vi "运维调试_质控单元.vi"() -> ()   [LabVIEW 2016, in "质控单元.lvlib"]
uses:
  <vilib>/Utility/miscctls.llb/LVPointTypeDef.ctl
  <vilib>/Analysis/6fits.llb/Curve Fitting Criteria.ctl
  <vilib>/Plasmionique/MB Master/MB_Master_Serial/MB_Master_Serial.lvclass
  D:/Program Files (x86)/National Instruments/LabVIEW 2016/vi.lib/Plasmionique/MB Master/MB_Master/MB_Master.lvclass
  <vilib>/Utility/config.llb/Read Key (I32).vi
  <vilib>/Utility/config.llb/Read Key (Double).vi
  <vilib>/Utility/config.llb/Read Key (Boolean).vi
  <vilib>/Utility/config.llb/Read Key (U32).vi
  <vilib>/Utility/config.llb/Write Key (I32).vi
  <vilib>/Utility/config.llb/Write Key (Double).vi
  <vilib>/Utility/config.llb/Write Key (Boolean).vi
  <vilib>/Utility/config.llb/Write Key (U32).vi
  <vilib>/Plasmionique/MB Master/MB Master.lvlib
  <vilib>/ptbypt/NI_PtbyPt.lvlib
  <vilib>/Utility/config.llb/NI_LVConfig.lvlib
  <vilib>/Analysis/NI_AALPro.lvlib
panel:
  in  "柱塞泵4":bool
  in  "CODCr量程选择":enum32{"H", "L", "AUTO"}(ring)
  in  "B 4":dbl caption="B4"
  in  "K 4":dbl caption="K4"
  out "通讯指示灯4":bool
  in  "CODCr选择":bool
  out "CODCr传感器故障报警":bool
  out "CODCr超时报警":bool
  out "CODMn超时报警":bool
  out "总磷总氮超时报警":bool
  out "氨氮进样超时报警":bool
  out "CODMn传感器故障报警":bool
  out "总磷总氮传感器故障报警":bool
  out "氨氮传感器故障报警":bool
  in  "CODCr加标回收启动":bool
  in  "CODCr停止":bool
  in  "CODCr排液":bool
  in  "CODCr调试":bool
  out "CODCr加标回收率":dbl caption="加标回收率" format="%.2f"
  out "CODCr加标体积":dbl caption="加标体积" format="%.3f"
  out "CODCr母液浓度":dbl caption="加标母液浓度" format="%.2f"
  out "CODCr加标水杯定容体积":dbl caption="加标水杯定容体积" format="%.2f"
  out "CODCr加标后水样浓度":dbl caption="加标后水样浓度" format="%.2f"
  out "CODCr加标前水样浓度":dbl caption="加标前水样浓度" format="%.2f"
  out "CODCr检出限":dbl caption="检出限" format="%.2f"
  out "CODCr量程":dbl caption="量程" format="%.2f"
  out "CODCr状态":u16(ring) caption="状态" items=["待机", "润洗", "进样", "等待取液", "排液"]
  out "质控流程中":bool
  out "CODMn质控中断报警":bool
  out "总磷质控中断报警":bool
  out "总氮质控中断报警":bool
  out "氨氮质控中断报警":bool
  in  "报警清除":bool
  in  "CODMn量程选择":enum32{"H", "L", "AUTO"}(ring)
  in  "CODMn加标回收启动":bool
  in  "总磷总氮加标回收启动":bool
  in  "氨氮加标回收启动":bool
  in  "总磷量程选择":enum32{"H", "L", "AUTO"}(ring)=enum."AUTO"
  in  "总氮量程选择":enum32{"H", "L", "AUTO"}(ring)=enum."AUTO"
  in  "氨氮量程选择":enum32{"H", "L", "AUTO"}(ring)=enum."AUTO"
  out "线性值":T1
  out "通讯指示灯3":bool
  out "通讯指示灯2":bool
  out "通讯指示灯1":bool
  in  "CODMn选择":bool
  in  "总磷总氮模块选择":bool
  in  "氨氮模块":bool
  in  "枚举":enum16{"柱塞泵1", "柱塞泵2", "柱塞泵3", "柱塞泵4"}(ring)
  in  "启用":bool
  in  "B 3":dbl caption="B3"
  in  "K 3":dbl caption="K3"
  in  "B 2":dbl caption="B2"
  in  "K 2":dbl caption="K2"
  in  "B":dbl caption="B1"
  in  "K":dbl caption="K1"
  out "r^2":dbl format="%_6g"
  out "拟合方程":string
  in  "实际体积 5":dbl
  in  "标准体积 5":dbl
  in  "实际体积 4":dbl
  in  "标准体积 4":dbl
  in  "实际体积 3":dbl
  in  "实际体积 2":dbl
  in  "实际体积 1":dbl
  in  "标准体积 3":dbl
  in  "标准体积 2":dbl
  in  "标准体积 1":dbl
  in  "读取":bool
  in  "柱塞泵3":bool
  in  "柱塞泵2":bool
  in  "柱塞泵1":bool
  in  "注出体积选择":u16(ring) items=["0.1mL", "0.3mL", "0.5mL", "0.8mL", "1.0mL"]
  out "Serial Config":T2={"baud rate (bps)"=115200, "stop bits"=10, "parity"=0, "flow control"=0, "timeout"=100, "retries"=1} {"stop bits" items=["1.0"=10, "1.5"=15, "2.0"=20]; "parity" items=["None", "Odd", "Even", "Mark", "Space"]; "flow control" items=["None", "XON/XOFF", "RTS/CTS", "XON/XOFF & RTS/CTS", "DTR/DSR", "XON/XOFF & DTR/DSR"]}
  out "VISA Resource":refnum<visa-resource-name>="COM8"
  in  "背隙补偿步数 3":i32 min=0 max=2000
  in  "背隙补偿步数 2":i32 min=0 max=2000
  in  "写入":bool
  in  "背隙补偿步数":i32 min=0 max=2000
  in  "总氮停止":bool
  in  "总氮排液":bool
  in  "总氮调试":bool
  out "总氮加标回收率":dbl caption="加标回收率" format="%.2f"
  out "总氮加标体积":dbl caption="加标体积" format="%.3f"
  out "总氮母液浓度":dbl caption="加标母液浓度" format="%.3f"
  out "总氮加标水杯定容体积":dbl caption="加标水杯定容体积" format="%.2f"
  out "总氮加标后水样浓度":dbl caption="加标后水样浓度" format="%.3f"
  out "总氮加标前水样浓度":dbl caption="加标前水样浓度" format="%.3f"
  out "总氮检出限":dbl caption="检出限" format="%.3f"
  out "总氮量程":dbl caption="量程" format="%.2f"
  out "总氮状态":u16(ring) caption="状态" items=["待机", "润洗", "进样", "等待取液", "排液"]
  in  "返回":bool
  in  "查看":bool
  out "直接启动":bool
  out "常规启动":bool
  out "columns":string[](array[string])
  out "data":T3
  out "COD平行样测完标志":bool
  out "氨氮总磷平行样测完标志":bool
  out "输出簇 2":T4
  out "常规启动 2":bool
  out "直接启动 2":bool
  out "启动模块 2":cluster{"氨氮1":bool, "总磷1":bool, " COD1":bool}
  in  "停止测量":bool
  in  "加标回收":bool
  in  "平行样测试":bool
  in  "CODMn停止":bool
  in  "CODMn排液":bool
  in  "CODMn调试":bool
  in  "总磷停止":bool
  in  "总磷排液":bool
  in  "总磷调试":bool
  out "COD加标回收率":dbl caption="加标回收率" format="%.2f"
  out "COD加标体积":dbl caption="加标体积" format="%.3f"
  out "COD母液浓度":dbl caption="加标母液浓度" format="%.2f"
  out "COD加标水杯定容体积":dbl caption="加标水杯定容体积" format="%.2f"
  out "COD加标后水样浓度":dbl caption="加标后水样浓度" format="%.2f"
  out "COD加标前水样浓度":dbl caption="加标前水样浓度" format="%.2f"
  out "COD检出限":dbl caption="检出限" format="%.2f"
  out "COD量程":dbl caption="量程" format="%.2f"
  out "CODMn状态":u16(ring) caption="状态" items=["待机", "润洗", "进样", "等待取液", "排液"]
  out "总磷加标回收率":dbl caption="加标回收率" format="%.2f"
  out "总磷加标体积":dbl caption="加标体积" format="%.3f"
  out "总磷母液浓度":dbl caption="加标母液浓度" format="%.3f"
  out "总磷加标水杯定容体积":dbl caption="加标水杯定容体积" format="%.2f"
  out "总磷加标后水样浓度":dbl caption="加标后水样浓度" format="%.3f"
  out "总磷加标前水样浓度":dbl caption="加标前水样浓度" format="%.3f"
  out "总磷检出限":dbl caption="检出限" format="%.3f"
  out "总磷量程":dbl caption="量程" format="%.2f"
  out "总磷状态":u16(ring) caption="状态" items=["待机", "润洗", "进样", "等待取液", "排液"]
  out "氨氮加标回收率":dbl caption="加标回收率" format="%.2f"
  out "氨氮加标体积":dbl caption="加标体积" format="%.3f"
  out "氨氮母液浓度":dbl caption="加标母液浓度" format="%.3f"
  out "氨氮加标水杯定容体积":dbl caption="加标水杯定容体积" format="%.2f"
  out "氨氮加标后水样浓度":dbl caption="加标后水样浓度" format="%.3f"
  out "氨氮加标前水样浓度":dbl caption="加标前水样浓度" format="%.3f"
  out "氨氮检出限":dbl caption="检出限" format="%.3f"
  out "氨氮量程":dbl caption="量程" format="%.2f"
  out "氨氮状态":u16(ring) caption="状态" items=["待机", "润洗", "进样", "等待取液", "排液"]
  in  "氨氮停止":bool
  in  "氨氮排液":bool
  in  "氨氮调试":bool
  # "状态显示区"
  # "参数配置区"
  # "2000步等于1mL\n100步等于0.05mL\n20步等于0.01mL\n2步等于0.001mL\n（初始默认100步）"
  # "辅助计算区"
  # "柱塞泵调试区"
  # "CODCr质控参数"
  # "%"
  # "mL"
  # "mg/L"
  # "mL"
  # "mg/L"
  # "mg/L"
  # "mg/L"
  # "mg/L"
  # "总氮质控参数"
  # "%"
  # "mL"
  # "mg/L"
  # "mL"
  # "mg/L"
  # "mg/L"
  # "mg/L"
  # "mg/L"
  # "CODMn质控参数"
  # "%"
  # "mL"
  # "mg/L"
  # "mL"
  # "mg/L"
  # "mg/L"
  # "mg/L"
  # "mg/L"
  # "总磷质控参数"
  # "%"
  # "mL"
  # "mg/L"
  # "mL"
  # "mg/L"
  # "mg/L"
  # "mg/L"
  # "mg/L"
  # "氨氮质控参数"
  # "%"
  # "mL"
  # "mg/L"
  # "mL"
  # "mg/L"
  # "mg/L"
  # "mg/L"
  # "mg/L"
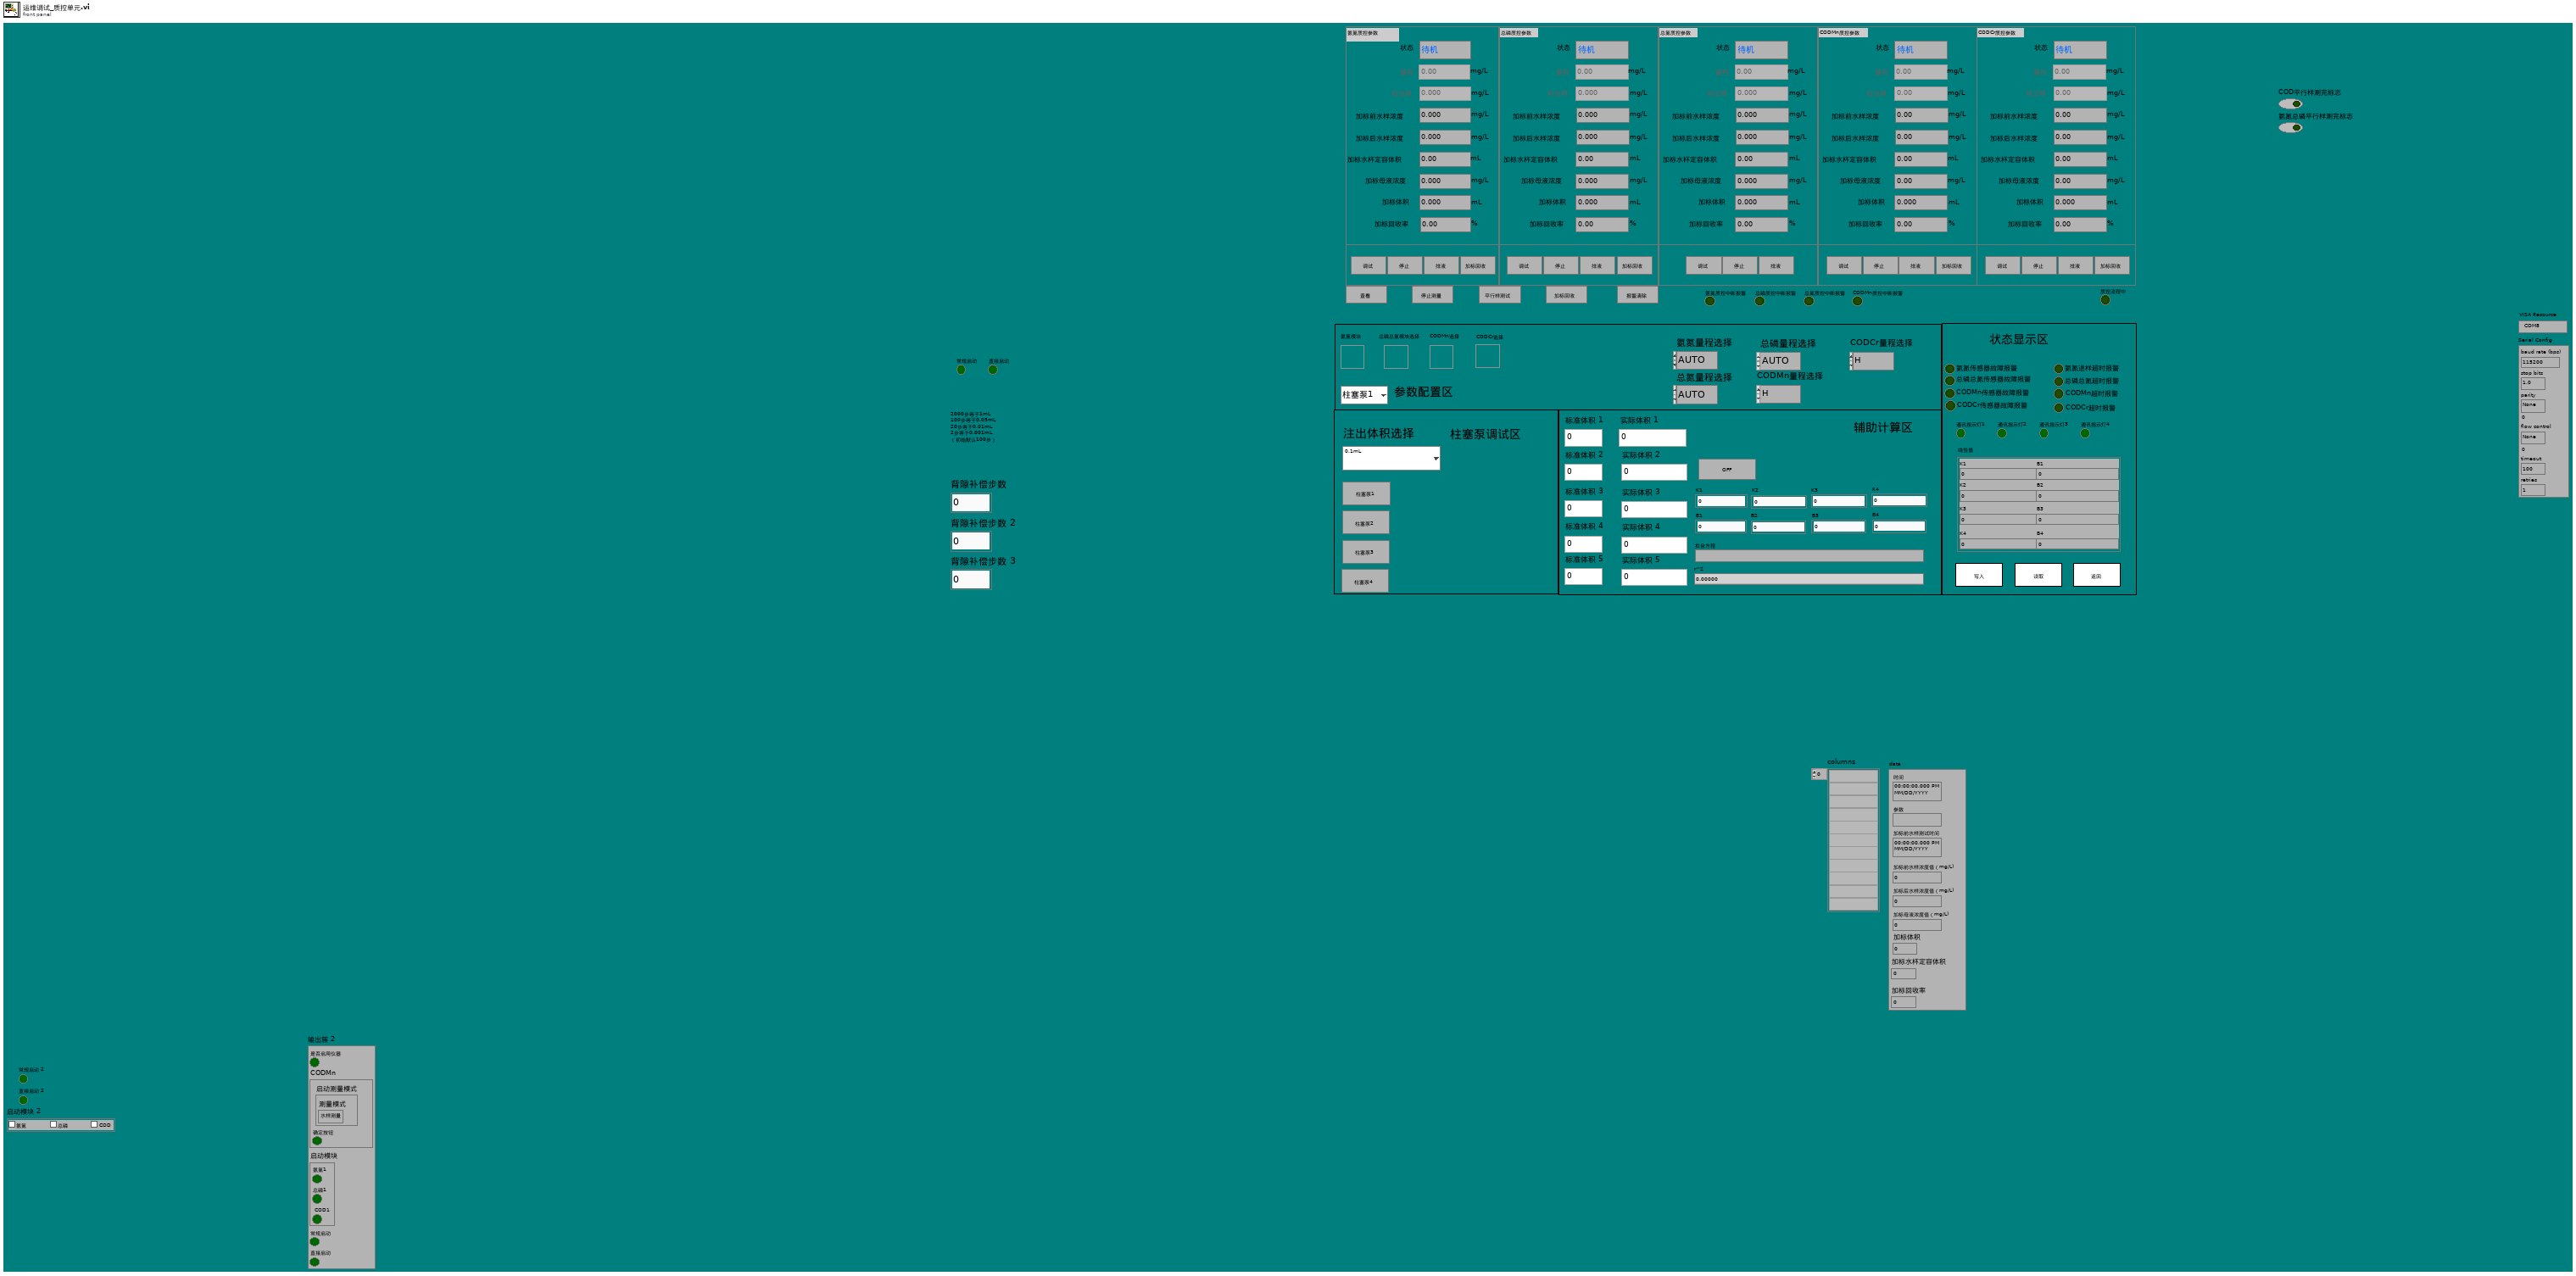
[diagram p1: front panel]
types:
  T1 = cluster{"K1":sgl, "B1":sgl, "K2":sgl, "B2":sgl, "K3":sgl, "B3":sgl, "K4":sgl, "B4":sgl}
  T2 = cluster{"baud rate (bps)":u32, "stop bits":u16, "parity":u16, "flow control":u16, "timeout":u32, "retries":i32}
  T3 = cluster{"时间":timestamp, "参数":string, "加标前水样测试时间":timestamp, "加标前水样浓度值（mg/L)":sgl, "加标后水样浓度值（mg/L)":sgl, "加标母液浓度值（mg/L)":sgl, "加标体积":dbl, "加标水杯定容体积":dbl, "加标回收率":dbl}
  T4 = cluster{"是否启用仪器":bool, "CODMn":cluster{"启动测量模式":cluster{"测量模式":enum16{"水样测量", "标样核查", "加标回收", "平行样", "校零", "校标"}}, "确定按钮":bool}, "启动模块":cluster{"氨氮1":bool, "总磷1":bool, " COD1":bool}, "常规启动":bool, "直接启动":bool}
  T5 = typedef "LVPointTypeDef.ctl" = cluster{"Horizontal":i16, "Vertical":i16}
  T6 = cluster{"量程":dbl, "检出限":dbl, "加标前水样浓度":dbl, "加标后水样浓度":dbl, "加标水杯定容体积":dbl, "加标母液浓度":dbl, "加标体积":dbl, "加标回收率":dbl}
  T7 = cluster{"因子编码":u32, "单位":u16, "标样参考值":sgl, "水样数据时间":timestamp, "水样实测值":sgl, "水样数据标识":string, "标样数据时间":timestamp, "标样实测值":sgl, "标样数据标识":string, "空白数据时间":timestamp, "空白实测值":sgl, "空白数据标识":string, "零点核查数据时间":timestamp, "零点核查实测值":sgl, "零点核查数据标识":string, "跨度核查数据时间":timestamp, "跨度核查实测值":sgl, "跨度核查数据标识":string, "加标回收数据时间":timestamp, "加标回收实测值":sgl, "加标回收数据标识":string, "平行样数据时间":timestamp, "平行样实测值":sgl, "平行样数据标识":string}
  T8 = cluster{"因子编码":u32, "单位":u16, "标样参考值":sgl, "水样数据时间":timestamp, "水样实测值":sgl, "水样数据标识":string, "标样数据时间":timestamp, "标样实测值":sgl, "标样数据标识":string, "空白数据时间":timestamp, "空白实测值":sgl, "空白数据标识":string, "零点核查数据时间":timestamp, "零点核查实测值":sgl, "零点核查数据标识":string, "跨度核查数据时间":timestamp, "跨度核查实测值":sgl, "跨度核查数据标识":string, "加标回收数据时间":timestamp, "加标回收实测值":sgl, "加标回收数据标识":string, "平行样数据时间":timestamp, "平行样实测值":sgl, "平行样数据标识":string, "F0":sgl, "F1":sgl, "F2":sgl, "F3":sgl, "F4":sgl, "F5":sgl, "F6":sgl, "F7":sgl, "温度":sgl, "湿度":sgl, "X值":sgl}
  T9 = enum8{"Enabled", "Disabled", "Disabled and Grayed Out"}
  T10 = typedef "NI_AALPro.lvlib/Curve Fitting Criteria.ctl" = u16
  T11 = typedef "NI_LVConfig.lvlib/Config Data RefNum.ctl" = refnum<k1>
  T12 = cluster{"是否启用仪器":bool, "CODMn":cluster{"启动测量模式":cluster{"测量模式":enum16{"水样测量", "标样核查", "加标回收", "平行样", "校零", "校标"}}, "确定按钮":bool}, "启动模块":cluster{"氨氮":bool, "总磷":bool, "总氮":bool, "CODMn":bool, "CODCr":bool}, "常规启动":bool, "直接启动":bool}
  T13 = cluster{"是否启用仪器":bool, "CODMn":cluster{"启动测量模式":cluster{"测量模式":enum16{"水样测量", "标样核查", "加标回收", "平行样", "校零", "校标"}}, "确定按钮":bool}, "启动模块":cluster{"氨氮":bool, "总磷":bool, "总氮":bool, "COD":bool}, "常规启动":bool, "直接启动":bool}
  T14 = cluster{"命令":string, cluster{"starting address":u16, "holding register value":u16}}
  T15 = cluster{"氨氮":bool, "总磷":bool, "总氮":bool, "CODMn":bool, "CODCr":bool}
  T16 = enum32{"Bad", "Idle", "Run top level", "Running"}
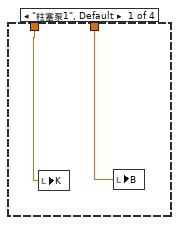
[diagram p3: hidden frame]
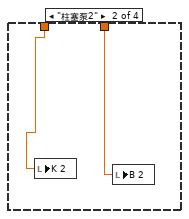
[diagram p4: hidden frame]
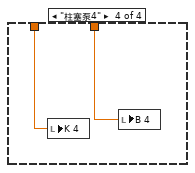
[diagram p5: hidden frame]
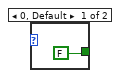
[diagram p8: hidden frame]
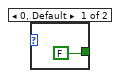
[diagram p9: hidden frame]
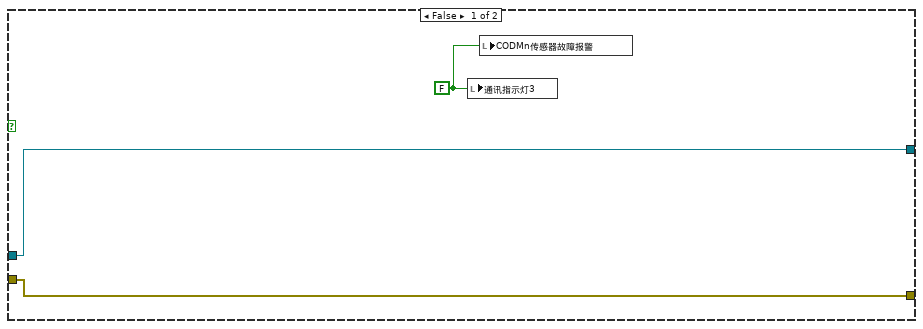
[diagram p10: hidden frame]
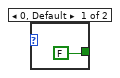
[diagram p11: hidden frame]
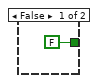
[diagram p12: hidden frame]
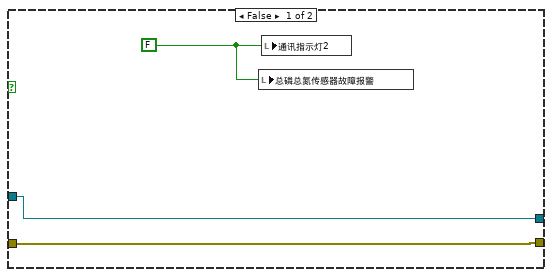
[diagram p13: hidden frame]
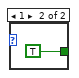
[diagram p14: hidden frame]
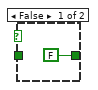
[diagram p15: hidden frame]
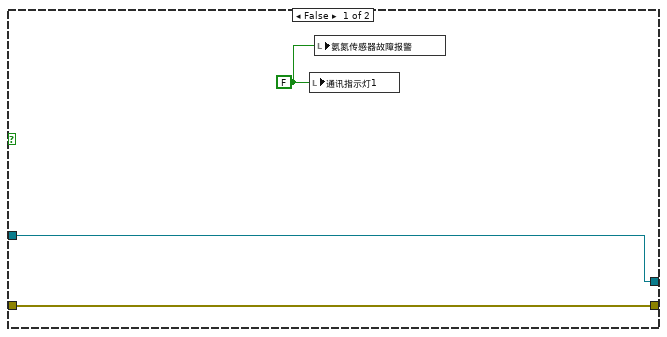
[diagram p16: hidden frame]
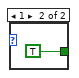
[diagram p17: hidden frame]
diagram:
  w21 = T2 {"baud rate (bps)"=115200, "stop bits"=10, "parity"=0, "flow control"=0, "timeout"=500, "retries"=1} ("Serial Config")
  w22 = refnum<visa-resource-name> "COM8" ("VISA Resource")
  n1 = global write "串口参数全局.vi" "Serial Config"(w21) -> ()
  n2 = control-ref of="总氮加标回收率"() -> (w36:refnum<vi>)
  n3 = control-ref of="总氮加标体积"() -> (w37:refnum<vi>)
  n4 = control-ref of="总氮加标水杯定容体积"() -> (w39:refnum<vi>)
  n5 = control-ref of="总氮加标后水样浓度"() -> (w40:refnum<vi>)
  n6 = control-ref of="总氮母液浓度"() -> (w38:refnum<vi>)
  n7 = global write "串口参数全局.vi" "VISA Resource"(w22) -> ()
  n8 = control-ref of="总氮检出限"() -> (w42:refnum<vi>)
  n9 = control-ref of="总氮加标前水样浓度"() -> (w41:refnum<vi>)
  n10 = control-ref of="总氮量程"() -> (w43:refnum<vi>)
  n11 = call <vilib>:"Open Serial Session.vi"("Mode (RTU)"=enum16{"RTU", "ASCII"}."RTU", "Slave ID"=u8 10, "Serial Config"=w21, "VISA Resource"=w22) -> ("Error out"=w54:errorcluster, "MB_Serial session"=w55:refnum<class "MB_Master_Serial.lvclass">)  [unwired: 6 in]
  n12 = control-ref of="COD加标水杯定容体积"() -> (w60:refnum<vi>)
  n13 = control-ref of="COD加标前水样浓度"() -> (w62:refnum<vi>)
  n14 = control-ref of="COD加标后水样浓度"() -> (w61:refnum<vi>)
  n15 = property on="窗格" class="Pane"("Origin"=T5 {"Horizontal"=0, "Vertical"=0} ("原点")) -> ()  [unwired: 2 in, 2 out]
  n16 = property on="窗格" class="Pane"("Origin"=T5 {"Horizontal"=0, "Vertical"=0} ("原点")) -> ()  [unwired: 2 in, 2 out]
  n17 = call "质控参数读取.vi"("section"="氨氮质控参数") -> ("error out"=w85:errorcluster, "参数"=w104:T6)  [unwired: 9 in]
  n18 = while {
    tunnel: w55 -> [w162]
    tunnel: w54 -> [w161]
    tunnel: [w128] -> w53
    tunnel: [w129] -> w23
    stop <- FALSE stop-if-true
    n19 = local read "CODCr加标前水样浓度"() -> (w126:dbl)
    n20 = global read "水样浓度全局.vi" "CODCr加标前水样浓度"() -> (w127:dbl)
    n21 = global read "质控测完标志全局 1.vi" "总磷总氮平行样测完标志"() -> (→"氨氮总磷平行样测完标志":bool)
    n22 = local read "氨氮模块"() -> (w135:bool)
    n23 = case shown="真" w135 {
      tunnel: w162 -> [w262 w282]
      tunnel: w161 -> [w261 w281]
      tunnel: [w262 w270] -> w139
      tunnel: [w261 w269] -> w137
      frame False {
        w260 = FALSE ("通讯指示灯1")
        n24 = local write "通讯指示灯1"(w260) -> ()
        n25 = local write "氨氮传感器故障报警"(w260) -> ()
      }
      frame True {
        n26 = property class="MB_Master_Serial"(reference=w282, "Properties:Slave ID"=u8 1 ("Slave ID")) -> (reference out=w277:refnum<class "MB_Master_Serial.lvclass">)  [unwired: 1 in, 1 out]
        n27 = call <vilib>:"Read Holding Registers.vi"("error in (no error)"=w281, "quantity"=u16 5, "starting address"=u16 100, "MB session in"=w277) -> ("error out"=w269:errorcluster, "Registers"=w278:u16[], "MB session out"=w270:refnum<class "MB_Master_Serial.lvclass">)  [unwired: 5 in]
        n28 = Index Array(array=w278, index #2=4 ("索引"), index #3=5 ("索引")) -> (element #1=w263:u16, element #2=w274:u16, element #3=w265:u16)  [unwired: 1 in]
        "氨氮状态" <- w263
        n29 = Unbundle By Name(w269) -> ("status"=w268:bool)
        n30 = case shown="0, 默认" w265 {
          tunnel: [FALSE TRUE] -> w264
          frame 0, Default {
          }
          frame 1 {
          }
        }
        "氨氮进样超时报警" <- w264
        n31 = global write "氨氮加标回收状态全局变量.vi" "氨氮状态"(w263) -> ()
        n32 = Not(x=w268) -> (.not. x?=→"通讯指示灯1":bool)
        n33 = Equal?(x=w274, y=u16 1) -> (x = y?=w271:bool)
        n34 = case shown="假" w271 {
          tunnel: w271 -> [_ w286]
          tunnel: [FALSE w286] -> w272
          frame False {
          }
          frame True {
          }
        }
        "氨氮传感器故障报警" <- w272
      }
    }
    n35 = global read "质控测完标志全局 1.vi" "氨氮加标回收测完标志"() -> (w148:bool)
    n36 = global read "质控测完标志全局 1.vi" "总磷加标回收测完标志"() -> (w140:bool)
    n37 = global read "质控测完标志全局 1.vi" "COD平行样测完标志"() -> (→"COD平行样测完标志":bool)
    n38 = global read "水样浓度全局.vi" "COD加标前水样浓度"() -> (w156:dbl)
    n39 = local read "总氮加标前水样浓度"() -> (w143:dbl)
    n40 = global read "水样浓度全局.vi" "氨氮加标前水样浓度"() -> (w160:dbl)
    n41 = global read "水样浓度全局.vi" "总磷加标前水样浓度"() -> (w158:dbl)
    n42 = local read "COD加标前水样浓度"() -> (w155:dbl)
    n43 = global read "水样浓度全局.vi" "总氮加标前水样浓度"() -> (w142:dbl)
    n44 = local read "氨氮加标前水样浓度"() -> (w159:dbl)
    n45 = local read "总磷加标前水样浓度"() -> (w157:dbl)
    n46 = global read "质控测完标志全局 1.vi" "COD加标回收测完标志"() -> (w123:bool)
    n47 = global read "质控测完标志全局 1.vi" "CODCr加标回收测完标志"() -> (w117:bool)
    n48 = global read "质控测完标志全局 1.vi" "总氮加标回收测完标志"() -> (w120:bool)
    n49 = Wait (ms)(milliseconds to wait=u32 1000 ("等待时间（毫秒）")) -> ()  [unwired: 1 out]
    n50 = Not Equal?(x=w127, y=w126) -> (x != y?=w125:bool)
    n51 = Not Equal?(x=w160, y=w159) -> (x != y?=w154:bool)
    n52 = Not Equal?(x=w158, y=w157) -> (x != y?=w152:bool)
    n53 = Not Equal?(x=w156, y=w155) -> (x != y?=w151:bool)
    n54 = Not Equal?(x=w142, y=w143) -> (x != y?=w141:bool)
    n55 = call <vilib>:"Boolean Crossing PtByPt.vi"("direction"=enum16{"either", "false-true", "true-false"}."false-true", "input"=w148) -> ("crossing"=w147:bool)  [unwired: 1 in]
    n56 = call <vilib>:"Boolean Crossing PtByPt.vi"("direction"=enum16{"either", "false-true", "true-false"}."false-true", "input"=w140) -> ("crossing"=w144:bool)  [unwired: 1 in]
    n57 = call <vilib>:"Boolean Crossing PtByPt.vi"("direction"=enum16{"either", "false-true", "true-false"}."false-true", "input"=w123) -> ("crossing"=w122:bool)  [unwired: 1 in]
    n58 = call <vilib>:"Boolean Crossing PtByPt.vi"("direction"=enum16{"either", "false-true", "true-false"}."false-true", "input"=w120) -> ("crossing"=w119:bool)  [unwired: 1 in]
    n59 = call <vilib>:"Boolean Crossing PtByPt.vi"("direction"=enum16{"either", "false-true", "true-false"}."false-true", "input"=w117) -> ("crossing"=w116:bool)  [unwired: 1 in]
    n60 = case shown="真" w147 {
      frame False {
      }
      frame True {
        n61 = flat-sequence {
          frame #0 {
            n62 = global read "VAR氨氮全局变量.vi" "测量数据区"() -> (w338:T7)
            n63 = Unbundle By Name(w338) -> ("加标回收实测值"=w339:sgl)
            n64 = property on="氨氮加标后水样浓度" class="DigNum (严格)"("Val(Sgnl)"=w339) -> ()  [unwired: 2 in, 2 out]
          }
          frame #1 {
            n65 = Wait (ms)(milliseconds to wait=u32 500 ("等待时间（毫秒）")) -> ()  [unwired: 1 out]
          }
          frame #2 {
            n66 = global read "VAR氨氮全局变量.vi" "测量数据区"() -> (w344:T7)
            n67 = local read "氨氮加标水杯定容体积"() -> (w350:dbl)
            n68 = global read "水样浓度全局.vi" "氨氮加标前水样浓度"() -> (w354:dbl)
            n69 = Unbundle By Name(w344) -> ("加标回收数据时间"=w347:timestamp)
            n70 = Unbundle By Name(w344) -> ("加标回收实测值"=w353:sgl)
            n71 = Unbundle By Name(w344) -> ("水样数据时间"=w345:timestamp)
            n72 = local read "氨氮加标回收率"() -> (w349:dbl)
            n73 = local read "氨氮母液浓度"() -> (w352:dbl)
            n74 = local read "氨氮加标体积"() -> (w351:dbl)
            n75 = Bundle By Name(cluster=T3 {"时间"=timestamp(0 s since 1904-01-01), "参数"="", "加标前水样测试时间"=timestamp(0 s since 1904-01-01), "加标前水样浓度值（mg/L)"=0.0, "加标后水样浓度值（mg/L)"=0.0, "加标母液浓度值（mg/L)"=0.0, "加标体积"=0.0, "加标水杯定容体积"=0.0, "加标回收率"=0.0} ("data"), "时间"=w347, "参数"="氨氮加标回收率" ("table"), "加标前水样测试时间"=w345, "加标前水样浓度值（mg/L)"=w354, "加标后水样浓度值（mg/L)"=w353, "加标母液浓度值（mg/L)"=w352, "加标体积"=w351, "加标水杯定容体积"=w350, "加标回收率"=w349) -> (w341:T3)
            n76 = local read "columns"() -> (w342:string[])
            n77 = local write "data"(w341) -> ()
            n78 = call "数据写入databaseZK.vi"("data"=w341, "columns"=w342, "table"="加标回收率") -> ()  [unwired: 8 in, 1 out]
          }
        }
      }
    }
    n79 = case shown="真" w144 {
      frame False {
      }
      frame True {
        n80 = flat-sequence {
          frame #0 {
            n81 = global read "VAR总磷总氮全局变量.vi" "总磷测量数据区"() -> (w321:T8)
            n82 = Unbundle By Name(w321) -> ("加标回收实测值"=w322:sgl)
            n83 = property on="总磷加标后水样浓度" class="DigNum (严格)"("Val(Sgnl)"=w322) -> ()  [unwired: 2 in, 2 out]
          }
          frame #1 {
            n84 = Wait (ms)(milliseconds to wait=u32 500 ("等待时间（毫秒）")) -> ()  [unwired: 1 out]
          }
          frame #2 {
            n85 = global read "VAR总磷总氮全局变量.vi" "总磷测量数据区"() -> (w327:T8)
            n86 = Unbundle By Name(w327) -> ("加标回收数据时间"=w330:timestamp)
            n87 = Unbundle By Name(w327) -> ("加标回收实测值"=w328:sgl)
            n88 = Unbundle By Name(w327) -> ("水样数据时间"=w329:timestamp)
            n89 = local read "总磷加标水杯定容体积"() -> (w334:dbl)
            n90 = local read "总磷加标回收率"() -> (w333:dbl)
            n91 = local read "总磷母液浓度"() -> (w336:dbl)
            n92 = local read "总磷加标体积"() -> (w335:dbl)
            n93 = global read "水样浓度全局.vi" "总磷加标前水样浓度"() -> (w337:dbl)
            n94 = Bundle By Name(cluster=T3 {"时间"=timestamp(0 s since 1904-01-01), "参数"="", "加标前水样测试时间"=timestamp(0 s since 1904-01-01), "加标前水样浓度值（mg/L)"=0.0, "加标后水样浓度值（mg/L)"=0.0, "加标母液浓度值（mg/L)"=0.0, "加标体积"=0.0, "加标水杯定容体积"=0.0, "加标回收率"=0.0} ("data"), "时间"=w330, "参数"="总磷加标回收率" ("table"), "加标前水样测试时间"=w329, "加标前水样浓度值（mg/L)"=w337, "加标后水样浓度值（mg/L)"=w328, "加标母液浓度值（mg/L)"=w336, "加标体积"=w335, "加标水杯定容体积"=w334, "加标回收率"=w333) -> (w324:T3)
            "data" <- w324
            n95 = local read "columns"() -> (w325:string[])
            n96 = call "数据写入databaseZK.vi"("data"=w324, "columns"=w325, "table"="加标回收率") -> ()  [unwired: 8 in, 1 out]
          }
        }
      }
    }
    n97 = case shown="真" w122 {
      frame False {
      }
      frame True {
        n98 = flat-sequence {
          frame #0 {
            n99 = global read "COD浓度全局变量.vi" "COD浓度（mg/L)"() -> (w306:dbl)
            n100 = property on="COD加标后水样浓度" class="DigNum (严格)"("Val(Sgnl)"=w306) -> ()  [unwired: 2 in, 2 out]
          }
          frame #1 {
            n101 = Wait (ms)(milliseconds to wait=u32 500 ("等待时间（毫秒）")) -> ()  [unwired: 1 out]
          }
          frame #2 {
            n102 = local read "COD加标水杯定容体积"() -> (w316:dbl)
            n103 = global read "水样浓度全局.vi" "COD加标前水样浓度"() -> (w320:dbl)
            n104 = global read "COD浓度全局变量.vi" "COD浓度（mg/L)"() -> (w319:dbl)
            n105 = global read "COD测量模式全局.vi" "加标回收启动时间"() -> (w312:timestamp)
            n106 = global read "COD测量模式全局.vi" "水样启动时间"() -> (w311:timestamp)
            n107 = local read "COD加标回收率"() -> (w315:dbl)
            n108 = local read "COD母液浓度"() -> (w318:dbl)
            n109 = local read "COD加标体积"() -> (w317:dbl)
            n110 = Bundle By Name(cluster=T3 {"时间"=timestamp(0 s since 1904-01-01), "参数"="", "加标前水样测试时间"=timestamp(0 s since 1904-01-01), "加标前水样浓度值（mg/L)"=0.0, "加标后水样浓度值（mg/L)"=0.0, "加标母液浓度值（mg/L)"=0.0, "加标体积"=0.0, "加标水杯定容体积"=0.0, "加标回收率"=0.0} ("data"), "时间"=w312, "参数"="CODMn加标回收率" ("table"), "加标前水样测试时间"=w311, "加标前水样浓度值（mg/L)"=w320, "加标后水样浓度值（mg/L)"=w319, "加标母液浓度值（mg/L)"=w318, "加标体积"=w317, "加标水杯定容体积"=w316, "加标回收率"=w315) -> (w308:T3)
            n111 = local read "columns"() -> (w309:string[])
            n112 = local write "data"(w308) -> ()
            n113 = call "数据写入databaseZK.vi"("data"=w308, "columns"=w309, "table"="加标回收率") -> ()  [unwired: 8 in, 1 out]
          }
        }
      }
    }
    n114 = case shown="真" w119 {
      frame False {
      }
      frame True {
        n115 = flat-sequence {
          frame #0 {
            n116 = global read "VAR总磷总氮全局变量.vi" "总氮测量数据区"() -> (w288:T8)
            n117 = Unbundle By Name(w288) -> ("加标回收实测值"=w287:sgl)
            n118 = property on="总氮加标后水样浓度" class="DigNum (严格)"("Val(Sgnl)"=w287) -> ()  [unwired: 2 in, 2 out]
          }
          frame #1 {
            n119 = Wait (ms)(milliseconds to wait=u32 500 ("等待时间（毫秒）")) -> ()  [unwired: 1 out]
          }
          frame #2 {
            n120 = global read "VAR总磷总氮全局变量.vi" "总氮测量数据区"() -> (w298:T8)
            n121 = global read "VAR总磷总氮全局变量.vi" "总氮测量数据区"() -> (w294:T8)
            n122 = global read "VAR总磷总氮全局变量.vi" "总氮测量数据区"() -> (w304:T8)
            n123 = local read "总氮加标水杯定容体积"() -> (w300:dbl)
            n124 = global read "水样浓度全局.vi" "总氮加标前水样浓度"() -> (w305:dbl)
            n125 = Unbundle By Name(w298) -> ("加标回收数据时间"=w295:timestamp)
            n126 = Unbundle By Name(w304) -> ("加标回收实测值"=w303:sgl)
            n127 = Unbundle By Name(w294) -> ("水样数据时间"=w293:timestamp)
            n128 = local read "总氮加标回收率"() -> (w299:dbl)
            n129 = local read "总氮母液浓度"() -> (w302:dbl)
            n130 = local read "总氮加标体积"() -> (w301:dbl)
            n131 = Bundle By Name(cluster=T3 {"时间"=timestamp(0 s since 1904-01-01), "参数"="", "加标前水样测试时间"=timestamp(0 s since 1904-01-01), "加标前水样浓度值（mg/L)"=0.0, "加标后水样浓度值（mg/L)"=0.0, "加标母液浓度值（mg/L)"=0.0, "加标体积"=0.0, "加标水杯定容体积"=0.0, "加标回收率"=0.0} ("data"), "时间"=w295, "参数"="总氮加标回收率" ("table"), "加标前水样测试时间"=w293, "加标前水样浓度值（mg/L)"=w305, "加标后水样浓度值（mg/L)"=w303, "加标母液浓度值（mg/L)"=w302, "加标体积"=w301, "加标水杯定容体积"=w300, "加标回收率"=w299) -> (w290:T3)
            n132 = local read "columns"() -> (w291:string[])
            n133 = local write "data"(w290) -> ()
            n134 = call "数据写入databaseZK.vi"("data"=w290, "columns"=w291, "table"="加标回收率") -> ()  [unwired: 8 in, 1 out]
          }
        }
      }
    }
    n135 = case shown="真" w116 {
      frame False {
      }
      frame True {
        n136 = flat-sequence {
          frame #0 {
            n137 = global read "CODcr全局变量.vi" "测量数据区"() -> (w166:T7)
            n138 = Unbundle By Name(w166) -> ("加标回收实测值"=w165:sgl)
            n139 = property on="CODCr加标后水样浓度" class="DigNum (严格)"("Val(Sgnl)"=w165) -> ()  [unwired: 2 in, 2 out]
          }
          frame #1 {
            n140 = Wait (ms)(milliseconds to wait=u32 500 ("等待时间（毫秒）")) -> ()  [unwired: 1 out]
          }
          frame #2 {
            n141 = global read "CODcr全局变量.vi" "测量数据区"() -> (w174:T7)
            n142 = global read "CODcr全局变量.vi" "测量数据区"() -> (w173:T7)
            n143 = global read "CODcr全局变量.vi" "测量数据区"() -> (w172:T7)
            n144 = local read "CODCr加标水杯定容体积"() -> (w169:dbl)
            n145 = local read "CODCr加标回收率"() -> (w168:dbl)
            n146 = local read "CODCr母液浓度"() -> (w171:dbl)
            n147 = local read "CODCr加标体积"() -> (w170:dbl)
            n148 = global read "水样浓度全局.vi" "CODCr加标前水样浓度"() -> (w183:dbl)
            n149 = Unbundle By Name(w172) -> ("加标回收数据时间"=w179:timestamp)
            n150 = Unbundle By Name(w174) -> ("加标回收实测值"=w182:sgl)
            n151 = Unbundle By Name(w173) -> ("水样数据时间"=w178:timestamp)
            n152 = Bundle By Name(cluster=T3 {"时间"=timestamp(0 s since 1904-01-01), "参数"="", "加标前水样测试时间"=timestamp(0 s since 1904-01-01), "加标前水样浓度值（mg/L)"=0.0, "加标后水样浓度值（mg/L)"=0.0, "加标母液浓度值（mg/L)"=0.0, "加标体积"=0.0, "加标水杯定容体积"=0.0, "加标回收率"=0.0} ("data"), "时间"=w179, "参数"="CODCr加标回收率" ("table"), "加标前水样测试时间"=w178, "加标前水样浓度值（mg/L)"=w183, "加标后水样浓度值（mg/L)"=w182, "加标母液浓度值（mg/L)"=w171, "加标体积"=w170, "加标水杯定容体积"=w169, "加标回收率"=w168) -> (w175:T3)
            n153 = local read "columns"() -> (w176:string[])
            n154 = local write "data"(w175) -> ()
            n155 = call "数据写入databaseZK.vi"("data"=w175, "columns"=w176, "table"="加标回收率") -> ()  [unwired: 8 in, 1 out]
          }
        }
      }
    }
    n156 = Compound Arithmetic op=OR ("复合运算")(w154, w152, w151, w141, w125) -> (w153:bool)
    n157 = case shown="真" w153 {
      frame False {
      }
      frame True {
        n158 = global read "水样浓度全局.vi" "CODCr加标前水样浓度"() -> (w355:dbl)
        n159 = property on="CODCr加标前水样浓度" class="DigNum (严格)"("Val(Sgnl)"=w355) -> ()  [unwired: 2 in, 2 out]
        n160 = global read "水样浓度全局.vi" "COD加标前水样浓度"() -> (w357:dbl)
        n161 = global read "水样浓度全局.vi" "总氮加标前水样浓度"() -> (w356:dbl)
        n162 = global read "水样浓度全局.vi" "总磷加标前水样浓度"() -> (w358:dbl)
        n163 = global read "水样浓度全局.vi" "氨氮加标前水样浓度"() -> (w359:dbl)
        n164 = property on="总氮加标前水样浓度" class="DigNum (严格)"("Val(Sgnl)"=w356) -> ()  [unwired: 2 in, 2 out]
        n165 = property on="COD加标前水样浓度" class="DigNum (严格)"("Val(Sgnl)"=w357) -> ()  [unwired: 2 in, 2 out]
        n166 = property on="总磷加标前水样浓度" class="DigNum (严格)"("Val(Sgnl)"=w358) -> ()  [unwired: 2 in, 2 out]
        n167 = property on="氨氮加标前水样浓度" class="DigNum (严格)"("Val(Sgnl)"=w359) -> ()  [unwired: 2 in, 2 out]
      }
    }
    n168 = local read "总磷总氮模块选择"() -> (w134:bool)
    n169 = case shown="真" w134 {
      tunnel: w139 -> [w236 w250]
      tunnel: [w236 w249] -> w138
      tunnel: w137 -> [w235 w248]
      tunnel: [w235 w246] -> w136
      frame False {
        w234 = FALSE ("通讯指示灯2")
        n170 = local write "总磷总氮传感器故障报警"(w234) -> ()
        n171 = local write "通讯指示灯2"(w234) -> ()
      }
      frame True {
        n172 = property class="MB_Master_Serial"(reference=w250, "Properties:Slave ID"=u8 2 ("Slave ID")) -> (reference out=w252:refnum<class "MB_Master_Serial.lvclass">)  [unwired: 1 in, 1 out]
        n173 = call <vilib>:"Read Holding Registers.vi"("error in (no error)"=w248, "quantity"=u16 5, "starting address"=u16 100, "MB session in"=w252) -> ("error out"=w246:errorcluster, "Registers"=w255:u16[], "MB session out"=w249:refnum<class "MB_Master_Serial.lvclass">)  [unwired: 5 in]
        n174 = Unbundle By Name(w246) -> ("status"=w247:bool)
        n175 = Index Array(array=w255, index #2=4 ("索引")) -> (element #1=w239:u16, element #2=w242:u16, element #3=w237:u16)  [unwired: 2 in]
        "总氮状态" <- w239
        "总磷状态" <- w239
        n176 = case shown="0, 默认" w237 {
          tunnel: [FALSE TRUE] -> w238
          frame 0, Default {
          }
          frame 1 {
          }
        }
        "总磷总氮超时报警" <- w238
        n177 = Not(x=w247) -> (.not. x?=→"通讯指示灯2":bool)
        n178 = Equal?(x=w242, y=u16 1) -> (x = y?=w240:bool)
        n179 = case shown="真" w240 {
          tunnel: w240 -> [_ w259]
          tunnel: [FALSE w259] -> w241
          frame False {
          }
          frame True {
          }
        }
        "总磷总氮传感器故障报警" <- w241
        n180 = global write "氨氮加标回收状态全局变量.vi" "总磷状态"(w239) -> ()
        n181 = global write "氨氮加标回收状态全局变量.vi" "总氮状态"(w239) -> ()
      }
    }
    n182 = local read "CODMn选择"() -> (w133:bool)
    n183 = case shown="真" w133 {
      tunnel: [w210 w225] -> w130
      tunnel: w138 -> [w210 w217]
      tunnel: w136 -> [w209 w216]
      tunnel: [w209 w214] -> w131
      frame False {
        w208 = FALSE ("通讯指示灯3")
        n184 = local write "通讯指示灯3"(w208) -> ()
        n185 = local write "CODMn传感器故障报警"(w208) -> ()
      }
      frame True {
        n186 = property class="MB_Master_Serial"(reference=w217, "Properties:Slave ID"=u8 3 ("Slave ID")) -> (reference out=w228:refnum<class "MB_Master_Serial.lvclass">)  [unwired: 1 in, 1 out]
        n187 = call <vilib>:"Read Holding Registers.vi"("error in (no error)"=w216, "quantity"=u16 5, "starting address"=u16 100, "MB session in"=w228) -> ("error out"=w214:errorcluster, "Registers"=w224:u16[], "MB session out"=w225:refnum<class "MB_Master_Serial.lvclass">)  [unwired: 5 in]
        n188 = Unbundle By Name(w214) -> ("status"=w215:bool)
        n189 = Index Array(array=w224, index #2=4 ("索引")) -> (element #1=w222:u16, element #2=w219:u16, element #3=w211:u16)  [unwired: 2 in]
        "CODMn状态" <- w222
        n190 = global write "氨氮加标回收状态全局变量.vi" "COD状态"(w222) -> ()
        n191 = Not(x=w215) -> (.not. x?=→"通讯指示灯3":bool)
        n192 = case shown="1" w211 {
          tunnel: [FALSE TRUE] -> w212
          frame 0, Default {
          }
          frame 1 {
          }
        }
        "CODMn超时报警" <- w212
        n193 = Equal?(x=w219, y=u16 1) -> (x = y?=w221:bool)
        n194 = case shown="真" w221 {
          tunnel: w221 -> [_ w233]
          tunnel: [FALSE w233] -> w218
          frame False {
          }
          frame True {
          }
        }
        "CODMn传感器故障报警" <- w218
      }
    }
    n195 = local read "CODCr选择"() -> (w132:bool)
    n196 = case shown="真" w132 {
      tunnel: w131 -> [w184 w202]
      tunnel: w130 -> [w185 w201]
      tunnel: [w185 w194] -> w129
      tunnel: [w184 w193] -> w128
      frame False {
      }
      frame True {
        n197 = property class="MB_Master_Serial"(reference=w201, error in=w202, "Properties:Slave ID"=u8 4 ("Slave ID")) -> (reference out=w196:refnum<class "MB_Master_Serial.lvclass">, error out=w195:errorcluster)
        n198 = call <vilib>:"Read Holding Registers.vi"("error in (no error)"=w195, "quantity"=u16 5, "starting address"=u16 100, "MB session in"=w196) -> ("error out"=w193:errorcluster, "Registers"=w198:u16[], "MB session out"=w194:refnum<class "MB_Master_Serial.lvclass">)  [unwired: 5 in]
        n199 = Unbundle By Name(w193) -> ("status"=w192:bool)
        n200 = Index Array(array=w198, index #2=4 ("索引")) -> (element #1=w190:u16, element #2=w187:u16, element #3=w189:u16)  [unwired: 2 in]
        "CODCr状态" <- w190
        n201 = global write "氨氮加标回收状态全局变量.vi" "CODCr状态"(w190) -> ()
        n202 = Not(x=w192) -> (.not. x?=→"通讯指示灯4":bool)
        n203 = case shown="1" w187 {
          tunnel: [FALSE TRUE] -> w186
          frame 0, Default {
          }
          frame 1 {
          }
        }
        "CODCr传感器故障报警" <- w186
        n204 = case shown="1" w189 {
          tunnel: [FALSE TRUE] -> w188
          frame 0, Default {
          }
          frame 1 {
          }
        }
        "CODCr超时报警" <- w188
      }
    }
  }
  n205 = Build Array(w43, w42, w41, w40, w39, w38, w37, w36) -> (w35:refnum<vi>[])
  n206 = while {
    stop <- FALSE stop-if-true
    n207 = global read "质控测完标志全局 1.vi" "氨氮质控流程中"() -> (w370:bool)
    n208 = global read "质控测完标志全局 1.vi" "COD质控流程中"() -> (w362:bool)
    n209 = global read "质控测完标志全局 1.vi" "总氮质控流程中"() -> (w366:bool)
    n210 = global read "质控中断报警全局.vi" "CODMn中断报警"() -> (→"CODMn质控中断报警":bool)
    n211 = global read "质控中断报警全局.vi" "氨氮中断报警"() -> (→"氨氮质控中断报警":bool)
    n212 = global read "质控中断报警全局.vi" "总氮中断报警"() -> (→"总氮质控中断报警":bool)
    n213 = Wait (ms)(milliseconds to wait=u32 100 ("等待时间（毫秒）")) -> ()  [unwired: 1 out]
    n214 = global read "质控中断报警全局.vi" "总磷中断报警"() -> (→"总磷质控中断报警":bool)
    n215 = local read "CODMn状态"() -> (w387:u16)
    n216 = global read "质控测完标志全局 1.vi" "质控流程中"() -> (w373:bool)
    "质控流程中" <- w373
    n217 = local read "总氮状态"() -> (w385:u16)
    n218 = local read "氨氮状态"() -> (w401:u16)
    n219 = local read "总磷状态"() -> (w392:u16)
    n220 = Not Equal To 0?(x=w385) -> (x != 0?=w384:bool)
    n221 = Not Equal To 0?(x=w401) -> (x != 0?=w400:bool)
    n222 = Not Equal To 0?(x=w392) -> (x != 0?=w394:bool)
    n223 = Not Equal To 0?(x=w387) -> (x != 0?=w391:bool)
    n224 = Select(t=T9."Disabled and Grayed Out" ("禁用"), s=w400, f=T9."Enabled") -> (s? t:f=w397:T9)
    n225 = Select(t=T9."Disabled and Grayed Out" ("禁用"), s=w394, f=T9."Enabled") -> (s? t:f=w393:T9)
    n226 = Select(t=T9."Disabled and Grayed Out" ("禁用"), s=w391, f=T9."Enabled") -> (s? t:f=w388:T9)
    n227 = Select(t=T9."Disabled and Grayed Out" ("禁用"), s=w370, f=T9."Enabled") -> (s? t:f=w368:T9)
    n228 = Select(t=T9."Disabled and Grayed Out" ("禁用"), s=w362, f=T9."Enabled") -> (s? t:f=w360:T9)
    n229 = Select(t=T9."Disabled and Grayed Out" ("禁用"), s=w366, f=T9."Enabled") -> (s? t:f=w364:T9)
    n230 = Select(t=T9."Disabled and Grayed Out" ("禁用"), s=w384, f=T9."Enabled") -> (s? t:f=w381:T9)
    n231 = Select(t=T9."Disabled and Grayed Out" ("禁用"), s=w373, f=T9."Enabled") -> (s? t:f=w372:T9)
    n232 = property on="氨氮加标回收启动" class="Bool"("DisabledEnum"=w368) -> ()  [unwired: 2 in, 2 out]
    n233 = property on="氨氮调试" class="Bool"("DisabledEnum"=w397) -> ()  [unwired: 2 in, 2 out]
    n234 = property on="总磷调试" class="Bool"("DisabledEnum"=w393) -> ()  [unwired: 2 in, 2 out]
    n235 = property on="COD调试" class="Bool"("DisabledEnum"=w388) -> ()  [unwired: 2 in, 2 out]
    n236 = property on="总磷总氮加标回收启动" class="Bool"("DisabledEnum"=w364) -> ()  [unwired: 2 in, 2 out]
    n237 = property on="CODMn加标回收启动" class="Bool"("DisabledEnum"=w360) -> ()  [unwired: 2 in, 2 out]
    n238 = property on="加标回收" class="Bool"("DisabledEnum"=w372) -> ()  [unwired: 2 in, 2 out]
    n239 = property on="总氮调试" class="Bool"("DisabledEnum"=w381) -> ()  [unwired: 2 in, 2 out]
    n240 = case shown="真" "启用" {
      frame False {
      }
      frame True {
        w419 = T10 0 items=["最小二乘", "最小绝对残差", "Bisquare"] ("method")
        n241 = Build Array("标准体积 1", "标准体积 2", "标准体积 3", "标准体积 4", "标准体积 5") -> (w416:dbl[])
        n242 = Build Array("实际体积 1", "实际体积 2", "实际体积 3", "实际体积 4", "实际体积 5") -> (w417:dbl[])
        n243 = call "线性公式质控用.vi"("标液浓度"=w416, "模型"=enum32{"线性", "多项式"}."线性", "监测浓度"=w417, "启用"=bool[] [TRUE, TRUE, TRUE, TRUE, TRUE], "method"=w419) -> ("拟合方程"=→"拟合方程":string, "r^2"=→"r^2":dbl, "slope"=w405:dbl, "intercept"=w404:dbl)  [unwired: 6 in, 1 out]
        n244 = case shown="\"柱塞泵3\"" "枚举" {
          tunnel: w405 -> [w423 w426 w427 w430]
          tunnel: w404 -> [w424 w425 w428 w429]
          frame "柱塞泵1", Default {
            n245 = local write "K"(w423) -> ()
            n246 = local write "B"(w424) -> ()
          }
          frame "柱塞泵2" {
            n247 = local write "K 2"(w426) -> ()
            n248 = local write "B 2"(w425) -> ()
          }
          frame "柱塞泵3" {
            n249 = local write "K 3"(w427) -> ()
            n250 = local write "B 3"(w428) -> ()
          }
          frame "柱塞泵4" {
            n251 = local write "K 4"(w430) -> ()
            n252 = local write "B 4"(w429) -> ()
          }
        }
      }
    }
  }
  n253 = control-ref of="总磷加标水杯定容体积"() -> (w69:refnum<vi>)
  n254 = control-ref of="氨氮加标水杯定容体积"() -> (w111:refnum<vi>)
  n255 = Unbundle By Name(w104) -> ("量程"=→"氨氮量程":dbl, "检出限"=→"氨氮检出限":dbl, "加标前水样浓度"=→"氨氮加标前水样浓度":dbl, "加标后水样浓度"=→"氨氮加标后水样浓度":dbl, "加标水杯定容体积"=→"氨氮加标水杯定容体积":dbl, "加标母液浓度"=→"氨氮母液浓度":dbl, "加标体积"=→"氨氮加标体积":dbl, "加标回收率"=→"氨氮加标回收率":dbl)
  n256 = control-ref of="总磷加标前水样浓度"() -> (w71:refnum<vi>)
  n257 = control-ref of="总磷加标后水样浓度"() -> (w70:refnum<vi>)
  n258 = control-ref of="氨氮加标前水样浓度"() -> (w112:refnum<vi>)
  n259 = control-ref of="氨氮加标后水样浓度"() -> (w108:refnum<vi>)
  n260 = control-ref of="COD加标回收率"() -> (w57:refnum<vi>)
  n261 = control-ref of="CODCr加标后水样浓度"() -> (w6:refnum<vi>)
  n262 = control-ref of="CODCr加标回收率"() -> (w2:refnum<vi>)
  n263 = control-ref of="CODCr加标前水样浓度"() -> (w7:refnum<vi>)
  n264 = control-ref of="CODCr加标水杯定容体积"() -> (w5:refnum<vi>)
  n265 = control-ref of="COD母液浓度"() -> (w59:refnum<vi>)
  n266 = control-ref of="COD加标体积"() -> (w58:refnum<vi>)
  n267 = control-ref of="CODCr检出限"() -> (w8:refnum<vi>)
  n268 = control-ref of="CODCr母液浓度"() -> (w4:refnum<vi>)
  n269 = control-ref of="CODCr量程"() -> (w9:refnum<vi>)
  n270 = control-ref of="CODCr加标体积"() -> (w3:refnum<vi>)
  n271 = call "质控参数读取.vi"("section"="总磷质控参数", "error in (no error)"=w85) -> ("error out"=w82:errorcluster, "参数"=w94:T6)  [unwired: 8 in]
  n272 = control-ref of="总磷加标回收率"() -> (w67:refnum<vi>)
  n273 = control-ref of="氨氮加标回收率"() -> (w106:refnum<vi>)
  n274 = control-ref of="COD检出限"() -> (w63:refnum<vi>)
  n275 = control-ref of="总磷母液浓度"() -> (w68:refnum<vi>)
  n276 = control-ref of="总磷加标体积"() -> (w66:refnum<vi>)
  n277 = control-ref of="氨氮母液浓度"() -> (w110:refnum<vi>)
  n278 = control-ref of="氨氮加标体积"() -> (w107:refnum<vi>)
  n279 = control-ref of="COD量程"() -> (w64:refnum<vi>)
  n280 = control-ref of="总磷检出限"() -> (w72:refnum<vi>)
  n281 = control-ref of="氨氮检出限"() -> (w113:refnum<vi>)
  n282 = control-ref of="总磷量程"() -> (w73:refnum<vi>)
  n283 = control-ref of="氨氮量程"() -> (w114:refnum<vi>)
  n284 = Build Array(w9, w8, w7, w6, w5, w4, w3, w2) -> (w1:refnum<vi>[])
  n285 = Obtain Notifier(name (unnamed)="采配水Process" ("名称（未命名）"), notification data type=FALSE) -> (notifier out=w48:refnum<notifier>)  [unwired: 2 in, 2 out]
  n286 = Build Array(w64, w63, w62, w61, w60, w59, w58, w57) -> (w56:refnum<vi>[])
  n287 = Build Array(w73, w72, w71, w70, w69, w68, w66, w67) -> (w65:refnum<vi>[])
  n288 = Build Array(w114, w113, w112, w108, w111, w110, w107, w106) -> (w109:refnum<vi>[])
  n289 = Unbundle By Name(w94) -> ("量程"=→"总磷量程":dbl, "检出限"=→"总磷检出限":dbl, "加标前水样浓度"=→"总磷加标前水样浓度":dbl, "加标后水样浓度"=→"总磷加标后水样浓度":dbl, "加标水杯定容体积"=→"总磷加标水杯定容体积":dbl, "加标母液浓度"=→"总磷母液浓度":dbl, "加标体积"=→"总磷加标体积":dbl, "加标回收率"=→"总磷加标回收率":dbl)
  n290 = call "质控参数读取.vi"("section"="COD质控参数", "error in (no error)"=w82) -> ("error out"=w33:errorcluster, "参数"=w84:T6)  [unwired: 8 in]
  n291 = Unbundle By Name(w84) -> ("量程"=→"COD量程":dbl, "检出限"=→"COD检出限":dbl, "加标前水样浓度"=→"COD加标前水样浓度":dbl, "加标后水样浓度"=→"COD加标后水样浓度":dbl, "加标水杯定容体积"=→"COD加标水杯定容体积":dbl, "加标母液浓度"=→"COD母液浓度":dbl, "加标体积"=→"COD加标体积":dbl, "加标回收率"=→"COD加标回收率":dbl)
  n292 = call "质控参数读取.vi"("section"="总氮质控参数", "error in (no error)"=w33) -> ("error out"=w18:errorcluster, "参数"=w32:T6)  [unwired: 8 in]
  n293 = Unbundle By Name(w32) -> ("量程"=→"总氮量程":dbl, "检出限"=→"总氮检出限":dbl, "加标前水样浓度"=→"总氮加标前水样浓度":dbl, "加标后水样浓度"=→"总氮加标后水样浓度":dbl, "加标水杯定容体积"=→"总氮加标水杯定容体积":dbl, "加标母液浓度"=→"总氮母液浓度":dbl, "加标体积"=→"总氮加标体积":dbl, "加标回收率"=→"总氮加标回收率":dbl)
  n294 = flat-sequence {
    frame #0 {
      w442 = "质控模块量程选择" ("section")
      w434 = "质控模块选择" ("section")
      w508 = "质控线性参数" ("section")
      w526 = "质控背隙补偿" ("section")
      n295 = call <vilib>:"Application Directory.vi"() -> ("Application Directory"=w532:path)
      n296 = Build Path(base path=w532, name or relative path="data\\Set.ini" ("名称或相对路径")) -> (appended path=w530:path)
      n297 = call <vilib>:"Open Config Data.vi"("configuration file path"=w530) -> ("error out"=w528:errorcluster, "refnum"=w529:T11)  [unwired: 8 in, 1 out]
      n298 = call-poly <vilib>:"Read Key.vi"("section"=w526, "error in (no error)"=w528, "key"="背隙值1", "refnum"=w529) -> ("error out"=w523:errorcluster, "value"=w518:i32, "refnum out"=w525:T11)  [unwired: 4 in, 1 out]
      n299 = local write "背隙补偿步数"(w518) -> ()
      n300 = call-poly <vilib>:"Read Key.vi"("section"=w526, "error in (no error)"=w523, "key"="背隙值2", "refnum"=w525) -> ("error out"=w521:errorcluster, "value"=w519:i32, "refnum out"=w522:T11)  [unwired: 4 in, 1 out]
      n301 = local write "背隙补偿步数 2"(w519) -> ()
      n302 = call-poly <vilib>:"Read Key.vi"("section"=w526, "error in (no error)"=w521, "key"="背隙值3", "refnum"=w522) -> ("error out"=w515:errorcluster, "value"=w517:i32, "refnum out"=w516:T11)  [unwired: 4 in, 1 out]
      n303 = local write "背隙补偿步数 3"(w517) -> ()
      n304 = call-poly <vilib>:"Read Key.vi"("section"=w508, "error in (no error)"=w515, "key"="标准体积1", "refnum"=w516) -> ("error out"=w511:errorcluster, "value"=w513:dbl, "refnum out"=w512:T11)  [unwired: 4 in, 1 out]
      n305 = local write "标准体积 1"(w513) -> ()
      n306 = call-poly <vilib>:"Read Key.vi"("section"=w508, "error in (no error)"=w511, "key"="标准体积2", "refnum"=w512) -> ("error out"=w509:errorcluster, "value"=w502:dbl, "refnum out"=w510:T11)  [unwired: 4 in, 1 out]
      n307 = local write "标准体积 2"(w502) -> ()
      n308 = call-poly <vilib>:"Read Key.vi"("section"=w508, "error in (no error)"=w509, "key"="标准体积3", "refnum"=w510) -> ("error out"=w506:errorcluster, "value"=w501:dbl, "refnum out"=w507:T11)  [unwired: 4 in, 1 out]
      n309 = local write "标准体积 3"(w501) -> ()
      n310 = call-poly <vilib>:"Read Key.vi"("section"=w508, "error in (no error)"=w506, "key"="标准体积4", "refnum"=w507) -> ("error out"=w504:errorcluster, "value"=w486:dbl, "refnum out"=w505:T11)  [unwired: 4 in, 1 out]
      n311 = local write "标准体积 4"(w486) -> ()
      n312 = Build Array("时间" ("table"), "参数" ("table"), "加标前水样测试时间" ("table"), "加标前水样浓度值" ("元素"), "加标后水样浓度值" ("元素"), "加标母液浓度值" ("元素"), "加标体积" ("元素"), "加标水杯定容体积" ("元素"), "加标回收率" ("元素")) -> (→"columns":string[])
      n313 = call-poly <vilib>:"Read Key.vi"("section"=w508, "error in (no error)"=w504, "key"="标准体积5", "refnum"=w505) -> ("error out"=w495:errorcluster, "value"=w485:dbl, "refnum out"=w496:T11)  [unwired: 4 in, 1 out]
      n314 = local write "标准体积 5"(w485) -> ()
      n315 = call-poly <vilib>:"Read Key.vi"("section"=w508, "error in (no error)"=w495, "key"="实际体积1", "refnum"=w496) -> ("error out"=w493:errorcluster, "value"=w484:dbl, "refnum out"=w494:T11)  [unwired: 4 in, 1 out]
      n316 = local write "实际体积 1"(w484) -> ()
      n317 = call-poly <vilib>:"Read Key.vi"("section"=w508, "error in (no error)"=w493, "key"="实际体积2", "refnum"=w494) -> ("error out"=w491:errorcluster, "value"=w483:dbl, "refnum out"=w492:T11)  [unwired: 4 in, 1 out]
      n318 = local write "实际体积 2"(w483) -> ()
      n319 = call-poly <vilib>:"Read Key.vi"("section"=w508, "error in (no error)"=w491, "key"="实际体积3", "refnum"=w492) -> ("error out"=w489:errorcluster, "value"=w480:dbl, "refnum out"=w490:T11)  [unwired: 4 in, 1 out]
      n320 = local write "实际体积 3"(w480) -> ()
      n321 = call-poly <vilib>:"Read Key.vi"("section"=w508, "error in (no error)"=w489, "key"="实际体积4", "refnum"=w490) -> ("error out"=w487:errorcluster, "value"=w479:dbl, "refnum out"=w488:T11)  [unwired: 4 in, 1 out]
      n322 = local write "实际体积 4"(w479) -> ()
      n323 = call-poly <vilib>:"Read Key.vi"("section"=w508, "error in (no error)"=w487, "key"="实际体积5", "refnum"=w488) -> ("error out"=w474:errorcluster, "value"=w478:dbl, "refnum out"=w475:T11)  [unwired: 4 in, 1 out]
      n324 = local write "实际体积 5"(w478) -> ()
      n325 = call-poly <vilib>:"Read Key.vi"("section"="质控手动体积选择", "error in (no error)"=w474, "key"="手动体积选择" ("section"), "refnum"=w475) -> ("error out"=w469:errorcluster, "value"=w471:i32, "refnum out"=w470:T11)  [unwired: 4 in, 1 out]
      n326 = local write "注出体积选择"(w471) -> ()
      n327 = call-poly <vilib>:"Read Key.vi"("section"=w434, "error in (no error)"=w469, "key"="模块1" ("section"), "refnum"=w470) -> ("error out"=w467:errorcluster, "value"=w459:bool, "refnum out"=w468:T11)  [unwired: 4 in, 1 out]
      n328 = call-poly <vilib>:"Read Key.vi"("section"=w434, "error in (no error)"=w467, "key"="模块2" ("section"), "refnum"=w468) -> ("error out"=w465:errorcluster, "value"=w460:bool, "refnum out"=w466:T11)  [unwired: 4 in, 1 out]
      n329 = local write "氨氮模块"(w459) -> ()
      n330 = local write "总磷总氮模块选择"(w460) -> ()
      n331 = call-poly <vilib>:"Read Key.vi"("section"=w434, "error in (no error)"=w465, "key"="模块3" ("section"), "refnum"=w466) -> ("error out"=w436:errorcluster, "value"=w461:bool, "refnum out"=w437:T11)  [unwired: 4 in, 1 out]
      n332 = local write "CODMn选择"(w461) -> ()
      n333 = call-poly <vilib>:"Read Key.vi"("section"=w434, "error in (no error)"=w436, "key"="模块4", "refnum"=w437) -> ("error out"=w432:errorcluster, "value"=w431:bool, "refnum out"=w433:T11)  [unwired: 4 in, 1 out]
      n334 = local write "CODCr选择"(w431) -> ()
      n335 = call-poly <vilib>:"Read Key.vi"("section"=w442, "error in (no error)"=w432, "key"="氨氮" ("section"), "refnum"=w433) -> ("error out"=w457:errorcluster, "value"=w448:u32, "refnum out"=w458:T11)  [unwired: 4 in, 1 out]
      n336 = local write "氨氮量程选择"(w448) -> ()
      n337 = call-poly <vilib>:"Read Key.vi"("section"=w442, "error in (no error)"=w457, "key"="总氮" ("section"), "refnum"=w458) -> ("error out"=w455:errorcluster, "value"=w447:u32, "refnum out"=w456:T11)  [unwired: 4 in, 1 out]
      n338 = local write "总氮量程选择"(w447) -> ()
      n339 = call-poly <vilib>:"Read Key.vi"("section"=w442, "error in (no error)"=w455, "key"="总磷" ("section"), "refnum"=w456) -> ("error out"=w453:errorcluster, "value"=w446:u32, "refnum out"=w454:T11)  [unwired: 4 in, 1 out]
      n340 = local write "总磷量程选择"(w446) -> ()
      n341 = call-poly <vilib>:"Read Key.vi"("section"=w442, "error in (no error)"=w453, "key"="CODMn" ("section"), "refnum"=w454) -> ("error out"=w443:errorcluster, "value"=w445:u32, "refnum out"=w444:T11)  [unwired: 4 in, 1 out]
      n342 = local write "CODMn量程选择"(w445) -> ()
      n343 = call-poly <vilib>:"Read Key.vi"("section"=w442, "error in (no error)"=w443, "key"="CODCr" ("section"), "refnum"=w444) -> ("error out"=w439:errorcluster, "value"=w440:u32, "refnum out"=w438:T11)  [unwired: 4 in, 1 out]
      n344 = local write "CODCr量程选择"(w440) -> ()
      n345 = call <vilib>:"Close Config Data.vi"("error in (no error)"=w439, "refnum"=w438) -> ()  [unwired: 8 in, 2 out]
    }
  }
  n346 = Obtain Queue(name (unnamed)="采配水" ("名称（未命名）"), element data type=cluster{"命令":string, "数据":variant} {"命令"="", "数据"=variant}) -> (queue out=w45:refnum<queue>)  [unwired: 3 in, 2 out]
  n347 = while {
    tunnel: w109 -> [w549]
    tunnel: w65 -> [w548]
    tunnel: w56 -> [w543]
    tunnel: w48 -> [w547]
    tunnel: w45 -> [w546]
    tunnel: w35 -> [w545]
    tunnel: w1 -> [w544]
    stop <- FALSE stop-if-true
    # "氨氮站号是1，总磷总氮站号是2，COD站号是3"
    n348 = event shown="[34] \"CODCr母液浓度\", \"CODCr加标水杯定容体积\", \"CODCr加标前水样浓度\", \"CODCr检出限\", \"CODCr量程\", \"CODCr加标后水样浓度\": 值改变" {
      selector: _ -> [_ _ _ _ _ _ _ _ _ _ _ _ _ _ _ _ _ _ _ _ _ _ _ _ _ _ _ _ _ _ _ _ _ _ _ _ _ _ _ _ _ _ _ _ _ _ _ _]
      dyn-events: _ -> [_ _ _ _ _ _ _ _ _ _ _ _ _ _ _ _ _ _ _ _ _ _ _ _ _ _ _ _ _ _ _ _ _ _ _ _ _ _ _ _ _ _ _ _ _ _ _ _]
      timeout: _ -> [_ _ _ _ _ _ _ _ _ _ _ _ _ _ _ _ _ _ _ _ _ _ _ _ _ _ _ _ _ _ _ _ _ _ _ _ _ _ _ _ _ _ _ _ _ _ _ _]
      tunnel: w549 -> [_ _ _ _ _ _ _ _ _ _ _ _ _ _ _ _ _ _ _ _ _ _ _ _ _ _ _ _ _ _ w916 _ _ _ _ w1013 _ _ _ _ _ _ _ _ _ _ _ _]
      tunnel: w548 -> [_ _ _ _ _ _ _ _ _ _ _ _ _ _ _ _ _ _ _ _ _ _ _ _ _ _ _ _ _ _ _ w930 _ _ _ w1010 _ _ _ _ _ _ _ _ _ _ _ _]
      tunnel: w543 -> [_ _ _ _ _ _ _ _ _ _ _ _ _ _ _ _ _ _ _ _ _ _ _ _ _ _ _ _ _ _ _ _ _ w968 _ w1009 _ _ _ _ _ _ _ _ _ _ _ _]
      tunnel: w547 -> [_ _ _ _ _ _ _ _ _ _ _ _ _ _ _ _ _ _ _ _ _ _ _ _ _ _ _ _ _ _ _ _ _ _ _ _ _ _ w1042 _ _ _ _ _ w1203 w1234 _ _]
      tunnel: w546 -> [_ _ _ _ _ _ _ _ _ _ _ _ _ _ _ _ _ _ _ _ _ _ _ _ _ _ _ _ _ _ _ _ _ _ _ _ _ _ _ _ _ _ _ _ _ w1231 _ _]
      tunnel: w545 -> [_ _ _ _ _ _ _ _ _ _ _ _ _ _ _ _ _ _ _ _ _ _ _ _ _ _ _ _ _ _ _ _ w948 _ _ w1006 _ _ _ _ _ _ _ _ _ _ _ _]
      tunnel: [_ _ _ _ _ _ _ _ _ _ _ _ _ _ _ _ _ _ _ _ _ _ _ _ _ w841 w882 w889 w896 w903 _ _ _ _ _ _ _ _ _ w1072 _ _ _ _ _ _ _ _] -> _
      tunnel: w544 -> [_ _ _ _ _ _ _ _ _ _ _ _ _ _ _ _ _ _ _ _ _ _ _ _ _ _ _ _ _ _ _ _ _ _ w986 w1005 _ _ _ _ _ _ _ _ _ _ _ _]
      event Timeout {
        n349 = event-data() -> ()  [unwired: 1 in, 3 out]
      }
      event "氨氮量程", "氨氮检出限", "氨氮加标前水样浓度", "氨氮加标水杯定容体积", "氨氮母液浓度", "氨氮加标后水样浓度": Mouse Down {
        n350 = event-data() -> ("CtlRef"=w554:refnum<vi>)  [unwired: 1 in, 7 out]
        n351 = property class="DigNum (严格)"(reference=w554) -> (reference out=w552:refnum<vi>, "Value"=w553:dbl)  [unwired: 1 in, 1 out]
        n352 = call "数字键盘.vi"("OldNumber"=w553) -> ("NewNumber"=w551:sgl)
        n353 = property class="DigNum (严格)"(reference=w552, "Val(Sgnl)"=w551) -> ()  [unwired: 1 in, 2 out]
      }
      event "总磷母液浓度", "总磷加标水杯定容体积", "总磷加标后水样浓度", "总磷加标前水样浓度", "总磷检出限", "总磷量程": Mouse Down {
        n354 = event-data() -> ("CtlRef"=w558:refnum<vi>)  [unwired: 1 in, 7 out]
        n355 = property class="DigNum (严格)"(reference=w558) -> (reference out=w556:refnum<vi>, "Value"=w557:dbl)  [unwired: 1 in, 1 out]
        n356 = call "数字键盘.vi"("OldNumber"=w557) -> ("NewNumber"=w555:sgl)
        n357 = property class="DigNum (严格)"(reference=w556, "Val(Sgnl)"=w555) -> ()  [unwired: 1 in, 2 out]
      }
      event "总氮母液浓度", "总氮加标水杯定容体积", "总氮加标后水样浓度", "总氮加标前水样浓度", "总氮检出限", "总氮量程": Mouse Down {
        n358 = event-data() -> ("CtlRef"=w562:refnum<vi>)  [unwired: 1 in, 7 out]
        n359 = property class="DigNum (严格)"(reference=w562) -> (reference out=w560:refnum<vi>, "Value"=w561:dbl)  [unwired: 1 in, 1 out]
        n360 = call "数字键盘.vi"("OldNumber"=w561) -> ("NewNumber"=w559:sgl)
        n361 = property class="DigNum (严格)"(reference=w560, "Val(Sgnl)"=w559) -> ()  [unwired: 1 in, 2 out]
      }
      event "COD母液浓度", "COD加标水杯定容体积", "COD加标后水样浓度", "COD加标前水样浓度", "COD检出限", "COD量程": Mouse Down {
        n362 = event-data() -> ("CtlRef"=w566:refnum<vi>)  [unwired: 1 in, 7 out]
        n363 = property class="DigNum (严格)"(reference=w566) -> (reference out=w564:refnum<vi>, "Value"=w565:dbl)  [unwired: 1 in, 1 out]
        n364 = call "数字键盘.vi"("OldNumber"=w565) -> ("NewNumber"=w563:sgl)
        n365 = property class="DigNum (严格)"(reference=w564, "Val(Sgnl)"=w563) -> ()  [unwired: 1 in, 2 out]
      }
      event "CODCr检出限", "CODCr量程", "CODCr加标前水样浓度", "CODCr加标后水样浓度", "CODCr加标水杯定容体积", "CODCr母液浓度": Mouse Down {
        n366 = event-data() -> ("CtlRef"=w567:refnum<vi>)  [unwired: 1 in, 7 out]
        n367 = property class="DigNum (严格)"(reference=w567) -> (reference out=w569:refnum<vi>, "Value"=w570:dbl)  [unwired: 1 in, 1 out]
        n368 = call "数字键盘.vi"("OldNumber"=w570) -> ("NewNumber"=w568:sgl)
        n369 = property class="DigNum (严格)"(reference=w569, "Val(Sgnl)"=w568) -> ()  [unwired: 1 in, 2 out]
      }
      event "背隙补偿步数": Mouse Down {
        n370 = event-data() -> ()  [unwired: 1 in, 8 out]
        n371 = local read "背隙补偿步数"() -> (w572:i32)
        n372 = call "数字键盘.vi"("OldNumber"=w572) -> ("NewNumber"=w571:sgl)
        n373 = local write "背隙补偿步数"(w571) -> ()
      }
      event "标准体积 1": Mouse Down {
        n374 = event-data() -> ()  [unwired: 1 in, 8 out]
        n375 = local read "标准体积 1"() -> (w574:dbl)
        n376 = call "数字键盘.vi"("OldNumber"=w574) -> ("NewNumber"=w573:sgl)
        n377 = local write "标准体积 1"(w573) -> ()
      }
      event "标准体积 2": Mouse Down {
        n378 = event-data() -> ()  [unwired: 1 in, 8 out]
        n379 = local read "标准体积 2"() -> (w576:dbl)
        n380 = call "数字键盘.vi"("OldNumber"=w576) -> ("NewNumber"=w575:sgl)
        n381 = local write "标准体积 2"(w575) -> ()
      }
      event "标准体积 3": Mouse Down {
        n382 = event-data() -> ()  [unwired: 1 in, 8 out]
        n383 = local read "标准体积 3"() -> (w578:dbl)
        n384 = call "数字键盘.vi"("OldNumber"=w578) -> ("NewNumber"=w577:sgl)
        n385 = local write "标准体积 3"(w577) -> ()
      }
      event "标准体积 4": Mouse Down {
        n386 = event-data() -> ()  [unwired: 1 in, 8 out]
        n387 = local read "标准体积 4"() -> (w580:dbl)
        n388 = call "数字键盘.vi"("OldNumber"=w580) -> ("NewNumber"=w579:sgl)
        n389 = local write "标准体积 4"(w579) -> ()
      }
      event "标准体积 5": Mouse Down {
        n390 = event-data() -> ()  [unwired: 1 in, 8 out]
        n391 = local read "标准体积 5"() -> (w582:dbl)
        n392 = call "数字键盘.vi"("OldNumber"=w582) -> ("NewNumber"=w581:sgl)
        n393 = local write "标准体积 5"(w581) -> ()
      }
      event "实际体积 1": Mouse Down {
        n394 = event-data() -> ()  [unwired: 1 in, 8 out]
        n395 = local read "实际体积 1"() -> (w584:dbl)
        n396 = call "数字键盘.vi"("OldNumber"=w584) -> ("NewNumber"=w583:sgl)
        n397 = local write "实际体积 1"(w583) -> ()
      }
      event "实际体积 2": Mouse Down {
        n398 = event-data() -> ()  [unwired: 1 in, 8 out]
        n399 = local read "实际体积 2"() -> (w586:dbl)
        n400 = call "数字键盘.vi"("OldNumber"=w586) -> ("NewNumber"=w585:sgl)
        n401 = local write "实际体积 2"(w585) -> ()
      }
      event "实际体积 3": Mouse Down {
        n402 = event-data() -> ()  [unwired: 1 in, 8 out]
        n403 = local read "实际体积 3"() -> (w588:dbl)
        n404 = call "数字键盘.vi"("OldNumber"=w588) -> ("NewNumber"=w587:sgl)
        n405 = local write "实际体积 3"(w587) -> ()
      }
      event "实际体积 4": Mouse Down {
        n406 = event-data() -> ()  [unwired: 1 in, 8 out]
        n407 = local read "实际体积 4"() -> (w590:dbl)
        n408 = call "数字键盘.vi"("OldNumber"=w590) -> ("NewNumber"=w589:sgl)
        n409 = local write "实际体积 4"(w589) -> ()
      }
      event "实际体积 5": Mouse Down {
        n410 = event-data() -> ()  [unwired: 1 in, 8 out]
        n411 = local read "实际体积 5"() -> (w592:dbl)
        n412 = call "数字键盘.vi"("OldNumber"=w592) -> ("NewNumber"=w591:sgl)
        n413 = local write "实际体积 5"(w591) -> ()
      }
      event "K", "B", "K 2", "B 2", "K 3", "B 3", "K 4", "B 4": Mouse Down {
        n414 = event-data() -> ("CtlRef"=w596:refnum<vi>)  [unwired: 1 in, 7 out]
        n415 = property class="DigNum (严格)"(reference=w596) -> (reference out=w593:refnum<vi>, "Value"=w595:dbl)  [unwired: 1 in, 1 out]
        n416 = call "数字键盘.vi"("OldNumber"=w595) -> ("NewNumber"=w594:sgl)
        n417 = property class="DigNum (严格)"(reference=w593, "Value"=w594) -> ()  [unwired: 1 in, 2 out]
      }
      event "背隙补偿步数 2": Mouse Down {
        n418 = event-data() -> ()  [unwired: 1 in, 8 out]
        n419 = local read "背隙补偿步数 2"() -> (w597:i32)
        n420 = call "数字键盘.vi"("OldNumber"=w597) -> ("NewNumber"=w598:sgl)
        n421 = local write "背隙补偿步数 2"(w598) -> ()
      }
      event "背隙补偿步数 3": Mouse Down {
        n422 = event-data() -> ()  [unwired: 1 in, 8 out]
        n423 = local read "背隙补偿步数 3"() -> (w600:i32)
        n424 = call "数字键盘.vi"("OldNumber"=w600) -> ("NewNumber"=w599:sgl)
        n425 = local write "背隙补偿步数 3"(w599) -> ()
      }
      event "背隙补偿步数", "背隙补偿步数 2", "背隙补偿步数 3", "标准体积 1", "标准体积 2", "标准体积 3", "标准体积 4", "标准体积 5", "实际体积 1", "实际体积 2", "实际体积 3", "实际体积 4", "实际体积 5": Value Change {
        w621 = "质控线性参数" ("section")
        w652 = "质控背隙补偿" ("section")
        n426 = event-data() -> ()  [unwired: 1 in, 6 out]
        n427 = call <vilib>:"Application Directory.vi"() -> ("Application Directory"=w659:path)
        n428 = Build Path(base path=w659, name or relative path="data\\Set.ini" ("名称或相对路径")) -> (appended path=w657:path)
        n429 = call <vilib>:"Open Config Data.vi"("configuration file path"=w657) -> ("error out"=w655:errorcluster, "refnum"=w656:T11)  [unwired: 8 in, 1 out]
        n430 = call-poly <vilib>:"Write Key.vi"("section"=w652, "error in (no error)"=w655, "value"="背隙补偿步数", "key"="背隙值1", "refnum"=w656) -> ("error out"=w646:errorcluster, "refnum out"=w649:T11)  [unwired: 4 in, 1 out]
        n431 = call-poly <vilib>:"Write Key.vi"("section"=w652, "error in (no error)"=w646, "value"="背隙补偿步数 2", "key"="背隙值2", "refnum"=w649) -> ("error out"=w647:errorcluster, "refnum out"=w648:T11)  [unwired: 4 in, 1 out]
        n432 = local read "标准体积 1"() -> (w619:dbl)
        n433 = call-poly <vilib>:"Write Key.vi"("section"=w652, "error in (no error)"=w647, "value"="背隙补偿步数 3", "key"="背隙值3", "refnum"=w648) -> ("error out"=w642:errorcluster, "refnum out"=w643:T11)  [unwired: 4 in, 1 out]
        n434 = local read "标准体积 2"() -> (w618:dbl)
        n435 = local read "标准体积 3"() -> (w616:dbl)
        n436 = call-poly <vilib>:"Write Key.vi"("section"=w621, "error in (no error)"=w642, "value"=w619, "key"="标准体积1", "refnum"=w643) -> ("error out"=w640:errorcluster, "refnum out"=w641:T11)  [unwired: 4 in, 1 out]
        n437 = local read "标准体积 4"() -> (w612:dbl)
        n438 = call-poly <vilib>:"Write Key.vi"("section"=w621, "error in (no error)"=w640, "value"=w618, "key"="标准体积2", "refnum"=w641) -> ("error out"=w638:errorcluster, "refnum out"=w639:T11)  [unwired: 4 in, 1 out]
        n439 = call-poly <vilib>:"Write Key.vi"("section"=w621, "error in (no error)"=w638, "value"=w616, "key"="标准体积3", "refnum"=w639) -> ("error out"=w636:errorcluster, "refnum out"=w637:T11)  [unwired: 4 in, 1 out]
        n440 = local read "标准体积 5"() -> (w611:dbl)
        n441 = call-poly <vilib>:"Write Key.vi"("section"=w621, "error in (no error)"=w636, "value"=w612, "key"="标准体积4", "refnum"=w637) -> ("error out"=w634:errorcluster, "refnum out"=w635:T11)  [unwired: 4 in, 1 out]
        n442 = local read "实际体积 1"() -> (w605:dbl)
        n443 = call-poly <vilib>:"Write Key.vi"("section"=w621, "error in (no error)"=w634, "value"=w611, "key"="标准体积5", "refnum"=w635) -> ("error out"=w632:errorcluster, "refnum out"=w633:T11)  [unwired: 4 in, 1 out]
        n444 = local read "实际体积 2"() -> (w604:dbl)
        n445 = call-poly <vilib>:"Write Key.vi"("section"=w621, "error in (no error)"=w632, "value"=w605, "key"="实际体积1", "refnum"=w633) -> ("error out"=w630:errorcluster, "refnum out"=w631:T11)  [unwired: 4 in, 1 out]
        n446 = local read "实际体积 3"() -> (w603:dbl)
        n447 = local read "实际体积 4"() -> (w602:dbl)
        n448 = call-poly <vilib>:"Write Key.vi"("section"=w621, "error in (no error)"=w630, "value"=w604, "key"="实际体积2", "refnum"=w631) -> ("error out"=w628:errorcluster, "refnum out"=w629:T11)  [unwired: 4 in, 1 out]
        n449 = local read "实际体积 5"() -> (w601:dbl)
        n450 = call-poly <vilib>:"Write Key.vi"("section"=w621, "error in (no error)"=w628, "value"=w603, "key"="实际体积3", "refnum"=w629) -> ("error out"=w626:errorcluster, "refnum out"=w627:T11)  [unwired: 4 in, 1 out]
        n451 = call-poly <vilib>:"Write Key.vi"("section"=w621, "error in (no error)"=w626, "value"=w602, "key"="实际体积4", "refnum"=w627) -> ("error out"=w624:errorcluster, "refnum out"=w625:T11)  [unwired: 4 in, 1 out]
        n452 = call-poly <vilib>:"Write Key.vi"("section"=w621, "error in (no error)"=w624, "value"=w601, "key"="实际体积5", "refnum"=w625) -> ("error out"=w622:errorcluster, "refnum out"=w623:T11)  [unwired: 4 in, 1 out]
        n453 = call <vilib>:"Close Config Data.vi"("error in (no error)"=w622, "refnum"=w623) -> ()  [unwired: 8 in, 2 out]
      }
      event "氨氮模块", "总磷总氮模块选择", "CODMn选择", "CODCr选择": Value Change {
        w663 = "质控模块选择" ("section")
        n454 = event-data() -> ()  [unwired: 1 in, 6 out]
        n455 = call <vilib>:"Application Directory.vi"() -> ("Application Directory"=w681:path)
        n456 = Build Path(base path=w681, name or relative path="data\\Set.ini" ("名称或相对路径")) -> (appended path=w679:path)
        n457 = local read "氨氮模块"() -> (w669:bool)
        n458 = call <vilib>:"Open Config Data.vi"("configuration file path"=w679) -> ("error out"=w677:errorcluster, "refnum"=w678:T11)  [unwired: 8 in, 1 out]
        n459 = local read "总磷总氮模块选择"() -> (w668:bool)
        n460 = call-poly <vilib>:"Write Key.vi"("section"=w663, "error in (no error)"=w677, "value"=w669, "key"="模块1" ("section"), "refnum"=w678) -> ("error out"=w675:errorcluster, "refnum out"=w676:T11)  [unwired: 4 in, 1 out]
        n461 = local read "CODMn选择"() -> (w667:bool)
        n462 = call-poly <vilib>:"Write Key.vi"("section"=w663, "error in (no error)"=w675, "value"=w668, "key"="模块2" ("section"), "refnum"=w676) -> ("error out"=w673:errorcluster, "refnum out"=w674:T11)  [unwired: 4 in, 1 out]
        n463 = local read "CODCr选择"() -> (w660:bool)
        n464 = call-poly <vilib>:"Write Key.vi"("section"=w663, "error in (no error)"=w673, "value"=w667, "key"="模块3" ("section"), "refnum"=w674) -> ("error out"=w664:errorcluster, "refnum out"=w665:T11)  [unwired: 4 in, 1 out]
        n465 = call-poly <vilib>:"Write Key.vi"("section"=w663, "error in (no error)"=w664, "value"=w660, "key"="模块4" ("section"), "refnum"=w665) -> ("error out"=w661:errorcluster, "refnum out"=w662:T11)  [unwired: 4 in, 1 out]
        n466 = call <vilib>:"Close Config Data.vi"("error in (no error)"=w661, "refnum"=w662) -> ()  [unwired: 8 in, 2 out]
      }
      event "氨氮量程选择", "总氮量程选择", "总磷量程选择", "CODMn量程选择", "CODCr量程选择": Value Change {
        w688 = "质控模块量程选择" ("section")
        n467 = event-data() -> ()  [unwired: 1 in, 6 out]
        n468 = call <vilib>:"Application Directory.vi"() -> ("Application Directory"=w707:path)
        n469 = Build Path(base path=w707, name or relative path="data\\Set.ini" ("名称或相对路径")) -> (appended path=w705:path)
        n470 = local read "氨氮量程选择"() -> (w692:enum32{"H", "L", "AUTO"})
        n471 = call <vilib>:"Open Config Data.vi"("configuration file path"=w705) -> ("error out"=w703:errorcluster, "refnum"=w704:T11)  [unwired: 8 in, 1 out]
        n472 = local read "总氮量程选择"() -> (w691:enum32{"H", "L", "AUTO"})
        n473 = call-poly <vilib>:"Write Key.vi"("section"=w688, "error in (no error)"=w703, "value"=w692, "key"="氨氮" ("section"), "refnum"=w704) -> ("error out"=w701:errorcluster, "refnum out"=w702:T11)  [unwired: 4 in, 1 out]
        n474 = local read "总磷量程选择"() -> (w690:enum32{"H", "L", "AUTO"})
        n475 = call-poly <vilib>:"Write Key.vi"("section"=w688, "error in (no error)"=w701, "value"=w691, "key"="总氮" ("section"), "refnum"=w702) -> ("error out"=w699:errorcluster, "refnum out"=w700:T11)  [unwired: 4 in, 1 out]
        n476 = local read "CODMn量程选择"() -> (w689:enum32{"H", "L", "AUTO"})
        n477 = call-poly <vilib>:"Write Key.vi"("section"=w688, "error in (no error)"=w699, "value"=w690, "key"="总磷" ("section"), "refnum"=w700) -> ("error out"=w694:errorcluster, "refnum out"=w695:T11)  [unwired: 4 in, 1 out]
        n478 = call-poly <vilib>:"Write Key.vi"("section"=w688, "error in (no error)"=w694, "value"=w689, "key"="CODMn" ("section"), "refnum"=w695) -> ("error out"=w684:errorcluster, "refnum out"=w687:T11)  [unwired: 4 in, 1 out]
        n479 = local read "CODCr量程选择"() -> (w682:enum32{"H", "L", "AUTO"})
        n480 = call-poly <vilib>:"Write Key.vi"("section"=w688, "error in (no error)"=w684, "value"=w682, "key"="CODCr" ("section"), "refnum"=w687) -> ("error out"=w685:errorcluster, "refnum out"=w686:T11)  [unwired: 4 in, 1 out]
        n481 = call <vilib>:"Close Config Data.vi"("error in (no error)"=w685, "refnum"=w686) -> ()  [unwired: 8 in, 2 out]
      }
      event "写入": Value Change {
        n482 = event-data() -> ()  [unwired: 1 in, 6 out]
        n483 = local read "枚举"() -> (w709:enum16{"柱塞泵1", "柱塞泵2", "柱塞泵3", "柱塞泵4"})
        n484 = case shown="\"柱塞泵4\"" w709 {
          tunnel: [w710 w722 w733 w745] -> w708
          frame "柱塞泵1", Default {
            n485 = local read "K"() -> (w714:dbl)
            n486 = local read "B"() -> (w715:dbl)
            n487 = local read "背隙补偿步数"() -> (w711:i32)
            n488 = Build Array(w714, w715) -> (w716:dbl[])
            n489 = call "浮点转CDAB整形ZK.vi"("浮点数"=w716) -> ("CDAB整形输出"=w718:u16[])  [unwired: 10 in]
            n490 = Build Array(w711) -> (w717:i32[])
            n491 = Insert Into Array(array=w717, index=0 ("索引"), new element=w718) -> (w720:i32[])
            n492 = call "写入参数.vi"("values"=w720, "starting address"=u16 1, "Slave ID"=u8 1) -> ("error out"=w710:errorcluster)  [unwired: 8 in]
          }
          frame "柱塞泵2" {
            n493 = local read "背隙补偿步数 2"() -> (w724:i32)
            n494 = local read "K 2"() -> (w727:dbl)
            n495 = local read "B 2"() -> (w726:dbl)
            n496 = Build Array(w727, w726) -> (w728:dbl[])
            n497 = call "浮点转CDAB整形ZK.vi"("浮点数"=w728) -> ("CDAB整形输出"=w729:u16[])  [unwired: 10 in]
            n498 = Build Array(w724) -> (w723:i32[])
            n499 = Insert Into Array(array=w723, index=0 ("索引"), new element=w729) -> (w731:i32[])
            n500 = call "写入参数.vi"("values"=w731, "starting address"=u16 1, "Slave ID"=u8 2) -> ("error out"=w722:errorcluster)  [unwired: 8 in]
          }
          frame "柱塞泵3" {
            n501 = local read "背隙补偿步数 3"() -> (w735:i32)
            n502 = local read "K 3"() -> (w739:dbl)
            n503 = local read "B 3"() -> (w740:dbl)
            n504 = Build Array(w739, w740) -> (w741:dbl[])
            n505 = call "浮点转CDAB整形ZK.vi"("浮点数"=w741) -> ("CDAB整形输出"=w742:u16[])  [unwired: 10 in]
            n506 = Build Array(w735) -> (w737:i32[])
            n507 = Insert Into Array(array=w737, index=0 ("索引"), new element=w742) -> (w736:i32[])
            n508 = call "写入参数.vi"("values"=w736, "starting address"=u16 1, "Slave ID"=u8 3) -> ("error out"=w733:errorcluster)  [unwired: 8 in]
          }
          frame "柱塞泵4" {
            n509 = local read "K 4"() -> (w750:dbl)
            n510 = local read "B 4"() -> (w751:dbl)
            n511 = Build Array(w750, w751) -> (w752:dbl[])
            n512 = call "浮点转CDAB整形ZK.vi"("浮点数"=w752) -> ("CDAB整形输出"=w753:u16[])  [unwired: 10 in]
            n513 = Build Array(0 ("背隙补偿步数")) -> (w748:i32[])
            n514 = Insert Into Array(array=w748, index=0 ("索引"), new element=w753) -> (w747:i32[])
            n515 = call "写入参数.vi"("values"=w747, "starting address"=u16 1, "Slave ID"=u8 4) -> ("error out"=w745:errorcluster)  [unwired: 8 in]
          }
        }
        n516 = case shown="无错误" w708 {
          frame No Error {
            n517 = One Button Dialog(message="写入成功" ("消息"), button name ("OK")="确定" ("按钮名称（“确定”）")) -> ()  [unwired: 1 out]
          }
          frame Error {
            n518 = One Button Dialog(message="写入失败" ("消息"), button name ("OK")="确定" ("按钮名称（“确定”）")) -> ()  [unwired: 1 out]
          }
        }
      }
      event "读取": Value Change {
        n519 = event-data() -> ()  [unwired: 1 in, 6 out]
        n520 = local read "氨氮模块"() -> (w765:bool)
        n521 = case shown="假" w765 {
          tunnel: [errorcluster {"status"=FALSE, "code"=0, "source"=""} ("error out") w797] -> w775
          tunnel: [w790 w794] -> w773
          tunnel: [w789 w793] -> w772
          frame False {
            n522 = local read "线性值"() -> (w791:T1)
            n523 = Unbundle By Name(w791) -> ("K3"=w790:sgl, "B3"=w789:sgl)
          }
          frame True {
            n524 = call "读取参数.vi"("Slave ID"=u8 1, "starting address"=u16 1, "quantity"=u16 4) -> ("values"=w796:u16[], "error out"=w797:errorcluster)  [unwired: 6 in]
            n525 = call "浮点CDAB转换质控.vi"("数组"=w796) -> ("数组 2"=w795:sgl[])  [unwired: 10 in]
            n526 = Index Array(array=w795) -> (element #1=w794:sgl, element #2=w793:sgl)  [unwired: 2 in]
          }
        }
        n527 = local read "总磷总氮模块选择"() -> (w766:bool)
        n528 = case shown="假" w766 {
          tunnel: w775 -> [w801 w812]
          tunnel: [w801 w811] -> w774
          tunnel: [w803 w808] -> w771
          tunnel: [w802 w807] -> w770
          frame False {
            n529 = local read "线性值"() -> (w804:T1)
            n530 = Unbundle By Name(w804) -> ("K3"=w803:sgl, "B3"=w802:sgl)
          }
          frame True {
            n531 = call "读取参数.vi"("Slave ID"=u8 2, "starting address"=u16 1, "quantity"=u16 4, "Error in"=w812) -> ("values"=w810:u16[], "error out"=w811:errorcluster)  [unwired: 5 in]
            n532 = call "浮点CDAB转换质控.vi"("数组"=w810) -> ("数组 2"=w809:sgl[])  [unwired: 10 in]
            n533 = Index Array(array=w809) -> (element #1=w808:sgl, element #2=w807:sgl)  [unwired: 2 in]
          }
        }
        n534 = local read "CODMn选择"() -> (w767:bool)
        n535 = case shown="假" w767 {
          tunnel: w774 -> [w814 w825]
          tunnel: [w816 w822] -> w769
          tunnel: [w815 w821] -> w768
          tunnel: [w814 w818] -> w763
          frame False {
            n536 = local read "线性值"() -> (w817:T1)
            n537 = Unbundle By Name(w817) -> ("K3"=w816:sgl, "B3"=w815:sgl)
          }
          frame True {
            n538 = call "读取参数.vi"("Slave ID"=u8 3, "starting address"=u16 1, "quantity"=u16 4, "Error in"=w825) -> ("values"=w824:u16[], "error out"=w818:errorcluster)  [unwired: 5 in]
            n539 = call "浮点CDAB转换质控.vi"("数组"=w824) -> ("数组 2"=w823:sgl[])  [unwired: 10 in]
            n540 = Index Array(array=w823) -> (element #1=w822:sgl, element #2=w821:sgl)  [unwired: 2 in]
          }
        }
        n541 = local read "CODCr选择"() -> (w761:bool)
        n542 = case shown="真" w761 {
          tunnel: w763 -> [w776 w787]
          tunnel: [w778 w784] -> w760
          tunnel: [w777 w783] -> w759
          tunnel: [w776 w780] -> w762
          frame False {
            n543 = local read "线性值"() -> (w779:T1)
            n544 = Unbundle By Name(w779) -> ("K4"=w778:sgl, "B4"=w777:sgl)
          }
          frame True {
            n545 = call "读取参数.vi"("Slave ID"=u8 4, "starting address"=u16 1, "quantity"=u16 4, "Error in"=w787) -> ("values"=w786:u16[], "error out"=w780:errorcluster)  [unwired: 5 in]
            n546 = call "浮点CDAB转换质控.vi"("数组"=w786) -> ("数组 2"=w785:sgl[])  [unwired: 10 in]
            n547 = Index Array(array=w785) -> (element #1=w784:sgl, element #2=w783:sgl)  [unwired: 2 in]
          }
        }
        n548 = Bundle By Name(cluster=T1 {"K1"=0.0, "B1"=0.0, "K2"=0.0, "B2"=0.0, "K3"=0.0, "B3"=0.0, "K4"=0.0, "B4"=0.0} ("线性值"), "K1"=w773, "B1"=w772, "K2"=w771, "B2"=w770, "K3"=w769, "B3"=w768, "K4"=w760, "B4"=w759) -> (→"线性值":T1)
        n549 = case shown="无错误" w762 {
          frame No Error {
            n550 = One Button Dialog(message="读取成功" ("消息"), button name ("OK")="确定" ("按钮名称（“确定”）")) -> ()  [unwired: 1 out]
          }
          frame Error {
            n551 = One Button Dialog(message="读取失败" ("消息"), button name ("OK")="确定" ("按钮名称（“确定”）")) -> ()  [unwired: 1 out]
          }
        }
      }
      event "注出体积选择": Value Change {
        n552 = event-data() -> ()  [unwired: 1 in, 6 out]
        n553 = case shown="0" "注出体积选择" {
          tunnel: [0.1 0.3 0.5 0.8 1.0] -> w851
          frame 0 {
          }
          frame 1 {
          }
          frame 2 {
          }
          frame 3 {
          }
          frame 4, Default {
          }
        }
        n554 = local read "氨氮模块"() -> (w838:bool)
        n555 = Build Array(w851) -> (w839:dbl[])
        n556 = call "浮点转CDAB整形ZK.vi"("浮点数"=w839) -> ("CDAB整形输出"=w832:u16[])  [unwired: 10 in]
        n557 = case shown="真" w838 {
          tunnel: [_ w863] -> w853
          tunnel: [u16 8 ("starting address") w862] -> w834
          tunnel: w832 -> [_ w861]
          frame False {
          }
          frame True {
            w862 = u16 8 ("starting address")
            n558 = call "写入参数.vi"("values"=w861, "starting address"=w862, "Slave ID"=u8 1) -> ("error out"=w863:errorcluster)  [unwired: 8 in]
          }
        }
        n559 = local read "总磷总氮模块选择"() -> (w837:bool)
        n560 = case shown="真" w837 {
          tunnel: w853 -> [w865 w869]
          tunnel: [w865 w868] -> w852
          tunnel: w834 -> [_ w867]
          tunnel: w832 -> [_ w866]
          frame False {
          }
          frame True {
            n561 = call "写入参数.vi"("Error in"=w869, "values"=w866, "starting address"=w867, "Slave ID"=u8 2) -> ("error out"=w868:errorcluster)  [unwired: 7 in]
          }
        }
        n562 = local read "CODMn选择"() -> (w836:bool)
        n563 = case shown="真" w836 {
          tunnel: w852 -> [w871 w875]
          tunnel: w834 -> [_ w874]
          tunnel: [w871 w873] -> w833
          tunnel: w832 -> [_ w872]
          frame False {
          }
          frame True {
            n564 = call "写入参数.vi"("Error in"=w875, "values"=w872, "starting address"=w874, "Slave ID"=u8 3) -> ("error out"=w873:errorcluster)  [unwired: 7 in]
          }
        }
        n565 = local read "CODCr选择"() -> (w835:bool)
        n566 = case shown="真" w835 {
          tunnel: w833 -> [w854 w858]
          tunnel: w834 -> [_ w857]
          tunnel: [w854 w856] -> w831
          tunnel: w832 -> [_ w855]
          frame False {
          }
          frame True {
            n567 = call "写入参数.vi"("Error in"=w858, "values"=w855, "starting address"=w857, "Slave ID"=u8 4) -> ("error out"=w856:errorcluster)  [unwired: 7 in]
          }
        }
        n568 = call <vilib>:"Application Directory.vi"() -> ("Application Directory"=w850:path)
        n569 = Build Path(base path=w850, name or relative path="data\\Set.ini" ("名称或相对路径")) -> (appended path=w848:path)
        n570 = call <vilib>:"Open Config Data.vi"("error in (no error)"=w831, "configuration file path"=w848) -> ("error out"=w844:errorcluster, "refnum"=w845:T11)  [unwired: 7 in, 1 out]
        n571 = call-poly <vilib>:"Write Key.vi"("section"="质控手动体积选择", "error in (no error)"=w844, "value"="注出体积选择", "key"="手动体积选择" ("section"), "refnum"=w845) -> ("error out"=w846:errorcluster, "refnum out"=w847:T11)  [unwired: 4 in, 1 out]
        n572 = call <vilib>:"Close Config Data.vi"("error in (no error)"=w846, "refnum"=w847) -> ("error out"=w841:errorcluster)  [unwired: 8 in, 1 out]
      }
      event "柱塞泵1": Value Change {
        n573 = event-data() -> ()  [unwired: 1 in, 6 out]
        n574 = Build Array("柱塞泵1") -> (w883:bool[])
        n575 = call "多个线圈写入.vi"("values"=w883, "starting address"=u16 2104, "Slave ID"=u8 1) -> ("error out"=w882:errorcluster)  [unwired: 8 in]
        n576 = case shown="错误" w882 {
          frame No Error {
          }
          frame Error {
            n577 = One Button Dialog(message="启动失败" ("消息"), button name ("OK")="确定" ("按钮名称（“确定”）")) -> ()  [unwired: 1 out]
          }
        }
      }
      event "柱塞泵2": Value Change {
        n578 = event-data() -> ()  [unwired: 1 in, 6 out]
        n579 = Build Array("柱塞泵2") -> (w891:bool[])
        n580 = call "多个线圈写入.vi"("values"=w891, "starting address"=u16 2104, "Slave ID"=u8 2) -> ("error out"=w889:errorcluster)  [unwired: 8 in]
        n581 = case shown="错误" w889 {
          frame No Error {
          }
          frame Error {
            n582 = One Button Dialog(message="启动失败" ("消息"), button name ("OK")="确定" ("按钮名称（“确定”）")) -> ()  [unwired: 1 out]
          }
        }
      }
      event "柱塞泵3": Value Change {
        n583 = event-data() -> ()  [unwired: 1 in, 6 out]
        n584 = Build Array("柱塞泵3") -> (w898:bool[])
        n585 = call "多个线圈写入.vi"("values"=w898, "starting address"=u16 2104, "Slave ID"=u8 3) -> ("error out"=w896:errorcluster)  [unwired: 8 in]
        n586 = case shown="无错误" w896 {
          frame No Error {
          }
          frame Error {
            n587 = One Button Dialog(message="启动失败" ("消息"), button name ("OK")="确定" ("按钮名称（“确定”）")) -> ()  [unwired: 1 out]
          }
        }
      }
      event "柱塞泵4": Value Change {
        n588 = event-data() -> ()  [unwired: 1 in, 6 out]
        n589 = Build Array("柱塞泵4") -> (w905:bool[])
        n590 = call "多个线圈写入.vi"("values"=w905, "starting address"=u16 2104, "Slave ID"=u8 4) -> ("error out"=w903:errorcluster)  [unwired: 8 in]
        n591 = case shown="无错误" w903 {
          frame No Error {
          }
          frame Error {
            n592 = One Button Dialog(message="启动失败" ("消息"), button name ("OK")="确定" ("按钮名称（“确定”）")) -> ()  [unwired: 1 out]
          }
        }
      }
      event "氨氮量程", "氨氮检出限", "氨氮加标前水样浓度", "氨氮母液浓度", "氨氮加标水杯定容体积", "氨氮加标后水样浓度": Value Change {
        n593 = event-data() -> ()  [unwired: 1 in, 6 out]
        n594 = for {
          tunnel: w916 -> [w928] mode=indexing
          tunnel: [w927] -> w925 mode=indexing
          n595 = property class="DigNum (严格)"(reference=w928) -> ("Value"=w927:dbl)  [unwired: 1 in, 2 out]
        }
        n596 = Index Array(array=w925) -> (element #1=w924:dbl, element #2=w923:dbl, element #3=w910:dbl, element #4=w922:dbl, element #5=w921:dbl, element #6=w919:dbl)  [unwired: 6 in]
        n597 = Bundle By Name(cluster=T6 {"量程"=0.0, "检出限"=0.0, "加标前水样浓度"=0.0, "加标后水样浓度"=0.0, "加标水杯定容体积"=0.0, "加标母液浓度"=0.0, "加标体积"=0.0, "加标回收率"=0.0} ("参数"), "量程"=w924, "检出限"=w923, "加标前水样浓度"=w910, "加标后水样浓度"=w922, "加标水杯定容体积"=w921, "加标母液浓度"=w919) -> (w918:T6)
        n598 = global write "水样浓度全局.vi" "氨氮加标前水样浓度"(w910) -> ()
        n599 = call "加标回收率计算.vi"("参数"=w918) -> ("参数 out"=w917:T6)  [unwired: 10 in]
        n600 = Index Array(array=w916, index #1=6 ("索引")) -> (element #1=w915:refnum<vi>, element #2=w913:refnum<vi>)  [unwired: 1 in]
        n601 = call "质控参数保存.vi"("section"="氨氮质控参数", "参数"=w917) -> ()  [unwired: 9 in, 1 out]
        n602 = Unbundle By Name(w917) -> ("加标体积"=w911:dbl, "加标回收率"=w912:dbl)
        n603 = property class="DigNum (严格)"(reference=w915, "Value"=w911) -> ()  [unwired: 1 in, 2 out]
        n604 = property class="DigNum (严格)"(reference=w913, "Value"=w912) -> ()  [unwired: 1 in, 2 out]
      }
      event "总磷母液浓度", "总磷加标水杯定容体积", "总磷加标后水样浓度", "总磷加标前水样浓度", "总磷检出限", "总磷量程": Value Change {
        n605 = event-data() -> ()  [unwired: 1 in, 6 out]
        n606 = for {
          tunnel: w930 -> [w947] mode=indexing
          tunnel: [w946] -> w944 mode=indexing
          n607 = property class="DigNum (严格)"(reference=w947) -> ("Value"=w946:dbl)  [unwired: 1 in, 2 out]
        }
        n608 = Index Array(array=w944) -> (element #1=w943:dbl, element #2=w942:dbl, element #3=w929:dbl, element #4=w941:dbl, element #5=w940:dbl, element #6=w938:dbl)  [unwired: 6 in]
        n609 = global write "水样浓度全局.vi" "总磷加标前水样浓度"(w929) -> ()
        n610 = Bundle By Name(cluster=T6 {"量程"=0.0, "检出限"=0.0, "加标前水样浓度"=0.0, "加标后水样浓度"=0.0, "加标水杯定容体积"=0.0, "加标母液浓度"=0.0, "加标体积"=0.0, "加标回收率"=0.0} ("参数"), "量程"=w943, "检出限"=w942, "加标前水样浓度"=w929, "加标后水样浓度"=w941, "加标水杯定容体积"=w940, "加标母液浓度"=w938) -> (w937:T6)
        n611 = call "加标回收率计算.vi"("参数"=w937) -> ("参数 out"=w936:T6)  [unwired: 10 in]
        n612 = Index Array(array=w930, index #1=6 ("索引")) -> (element #1=w935:refnum<vi>, element #2=w932:refnum<vi>)  [unwired: 1 in]
        n613 = call "质控参数保存.vi"("section"="总磷质控参数", "参数"=w936) -> ()  [unwired: 9 in, 1 out]
        n614 = Unbundle By Name(w936) -> ("加标体积"=w933:dbl, "加标回收率"=w931:dbl)
        n615 = property class="DigNum (严格)"(reference=w935, "Value"=w933) -> ()  [unwired: 1 in, 2 out]
        n616 = property class="DigNum (严格)"(reference=w932, "Value"=w931) -> ()  [unwired: 1 in, 2 out]
      }
      event "总氮量程", "总氮检出限", "总氮加标前水样浓度", "总氮加标后水样浓度", "总氮加标水杯定容体积", "总氮母液浓度": Value Change {
        n617 = event-data() -> ()  [unwired: 1 in, 6 out]
        n618 = for {
          tunnel: w948 -> [w966] mode=indexing
          tunnel: [w965] -> w963 mode=indexing
          n619 = property class="DigNum (严格)"(reference=w966) -> ("Value"=w965:dbl)  [unwired: 1 in, 2 out]
        }
        n620 = Index Array(array=w963) -> (element #1=w962:dbl, element #2=w961:dbl, element #3=w949:dbl, element #4=w960:dbl, element #5=w959:dbl, element #6=w957:dbl)  [unwired: 6 in]
        n621 = global write "水样浓度全局.vi" "总氮加标前水样浓度"(w949) -> ()
        n622 = Bundle By Name(cluster=T6 {"量程"=0.0, "检出限"=0.0, "加标前水样浓度"=0.0, "加标后水样浓度"=0.0, "加标水杯定容体积"=0.0, "加标母液浓度"=0.0, "加标体积"=0.0, "加标回收率"=0.0} ("参数"), "量程"=w962, "检出限"=w961, "加标前水样浓度"=w949, "加标后水样浓度"=w960, "加标水杯定容体积"=w959, "加标母液浓度"=w957) -> (w956:T6)
        n623 = call "加标回收率计算.vi"("参数"=w956) -> ("参数 out"=w955:T6)  [unwired: 10 in]
        n624 = Index Array(array=w948, index #1=6 ("索引")) -> (element #1=w954:refnum<vi>, element #2=w951:refnum<vi>)  [unwired: 1 in]
        n625 = call "质控参数保存.vi"("section"="总氮质控参数", "参数"=w955) -> ()  [unwired: 9 in, 1 out]
        n626 = Unbundle By Name(w955) -> ("加标体积"=w952:dbl, "加标回收率"=w950:dbl)
        n627 = property class="DigNum (严格)"(reference=w954, "Value"=w952) -> ()  [unwired: 1 in, 2 out]
        n628 = property class="DigNum (严格)"(reference=w951, "Value"=w950) -> ()  [unwired: 1 in, 2 out]
      }
      event "COD母液浓度", "COD加标水杯定容体积", "COD加标后水样浓度", "COD加标前水样浓度", "COD检出限", "COD量程": Value Change {
        n629 = event-data() -> ()  [unwired: 1 in, 6 out]
        n630 = for {
          tunnel: w968 -> [w985] mode=indexing
          tunnel: [w984] -> w982 mode=indexing
          n631 = property class="DigNum (严格)"(reference=w985) -> ("Value"=w984:dbl)  [unwired: 1 in, 2 out]
        }
        n632 = Index Array(array=w982) -> (element #1=w981:dbl, element #2=w980:dbl, element #3=w967:dbl, element #4=w979:dbl, element #5=w978:dbl, element #6=w976:dbl)  [unwired: 6 in]
        n633 = global write "水样浓度全局.vi" "COD加标前水样浓度"(w967) -> ()
        n634 = Bundle By Name(cluster=T6 {"量程"=0.0, "检出限"=0.0, "加标前水样浓度"=0.0, "加标后水样浓度"=0.0, "加标水杯定容体积"=0.0, "加标母液浓度"=0.0, "加标体积"=0.0, "加标回收率"=0.0} ("参数"), "量程"=w981, "检出限"=w980, "加标前水样浓度"=w967, "加标后水样浓度"=w979, "加标水杯定容体积"=w978, "加标母液浓度"=w976) -> (w975:T6)
        n635 = call "加标回收率计算.vi"("参数"=w975) -> ("参数 out"=w974:T6)  [unwired: 10 in]
        n636 = Index Array(array=w968, index #1=6 ("索引")) -> (element #1=w973:refnum<vi>, element #2=w970:refnum<vi>)  [unwired: 1 in]
        n637 = call "质控参数保存.vi"("section"="COD质控参数", "参数"=w974) -> ()  [unwired: 9 in, 1 out]
        n638 = Unbundle By Name(w974) -> ("加标体积"=w971:dbl, "加标回收率"=w969:dbl)
        n639 = property class="DigNum (严格)"(reference=w973, "Value"=w971) -> ()  [unwired: 1 in, 2 out]
        n640 = property class="DigNum (严格)"(reference=w970, "Value"=w969) -> ()  [unwired: 1 in, 2 out]
      }
      event "CODCr母液浓度", "CODCr加标水杯定容体积", "CODCr加标前水样浓度", "CODCr检出限", "CODCr量程", "CODCr加标后水样浓度": Value Change {
        n641 = event-data() -> ()  [unwired: 1 in, 6 out]
        n642 = for {
          tunnel: w986 -> [w1004] mode=indexing
          tunnel: [w1003] -> w1001 mode=indexing
          n643 = property class="DigNum (严格)"(reference=w1004) -> ("Value"=w1003:dbl)  [unwired: 1 in, 2 out]
        }
        n644 = Index Array(array=w1001) -> (element #1=w1000:dbl, element #2=w999:dbl, element #3=w987:dbl, element #4=w998:dbl, element #5=w997:dbl, element #6=w995:dbl)  [unwired: 6 in]
        n645 = global write "水样浓度全局.vi" "CODCr加标前水样浓度"(w987) -> ()
        n646 = Bundle By Name(cluster=T6 {"量程"=0.0, "检出限"=0.0, "加标前水样浓度"=0.0, "加标后水样浓度"=0.0, "加标水杯定容体积"=0.0, "加标母液浓度"=0.0, "加标体积"=0.0, "加标回收率"=0.0} ("参数"), "量程"=w1000, "检出限"=w999, "加标前水样浓度"=w987, "加标后水样浓度"=w998, "加标水杯定容体积"=w997, "加标母液浓度"=w995) -> (w994:T6)
        n647 = call "加标回收率计算.vi"("参数"=w994) -> ("参数 out"=w993:T6)  [unwired: 10 in]
        n648 = Index Array(array=w986, index #1=6 ("索引")) -> (element #1=w992:refnum<vi>, element #2=w989:refnum<vi>)  [unwired: 1 in]
        n649 = call "质控参数保存.vi"("section"="CODCr质控参数", "参数"=w993) -> ()  [unwired: 9 in, 1 out]
        n650 = Unbundle By Name(w993) -> ("加标体积"=w990:dbl, "加标回收率"=w988:dbl)
        n651 = property class="DigNum (严格)"(reference=w992, "Value"=w990) -> ()  [unwired: 1 in, 2 out]
        n652 = property class="DigNum (严格)"(reference=w989, "Value"=w988) -> ()  [unwired: 1 in, 2 out]
      }
      event "氨氮调试", "总磷调试", "CODMn调试", "总氮调试", "CODCr调试": Value Change {
        n653 = event-data() -> ("CtlRef"=w1012:refnum<vi>)  [unwired: 1 in, 5 out]
        n654 = property class="Bool"(reference=w1012) -> ("Label.Text"=w1011:string)  [unwired: 1 in, 2 out]
        n655 = case shown="\"CODCr调试\"" w1011 {
          tunnel: w1013 -> [w1014 _ _ _ _]
          tunnel: w1010 -> [_ w1016 _ _ _]
          tunnel: w1009 -> [_ _ _ w1020 _]
          tunnel: ["氨氮模块" ("标题") "总磷模块" ("标题") "总氮模块" ("标题") "CODMn模块" ("标题") "CODCr模块" ("标题")] -> w1008
          tunnel: [w1014 w1016 w1018 w1020 w1022] -> w1007
          tunnel: w1006 -> [_ _ w1018 _ _]
          tunnel: w1005 -> [_ _ _ _ w1022]
          frame "氨氮调试", Default {
          }
          frame "总磷调试" {
          }
          frame "总氮调试" {
          }
          frame "CODMn调试" {
          }
          frame "CODCr调试" {
          }
        }
        n656 = call "加标模块单控对话框.vi"("数组"=w1007, "标题"=w1008) -> ()  [unwired: 10 in]
      }
      event "氨氮停止", "总磷停止", "CODMn停止", "总氮停止", "CODCr停止": Value Change {
        n657 = event-data() -> ("CtlRef"=w1028:refnum<vi>)  [unwired: 1 in, 5 out]
        n658 = property class="Bool"(reference=w1028) -> ("Label.Text"=w1027:string)  [unwired: 1 in, 2 out]
        n659 = case shown="\"CODCr模块\"" w1027 {
          tunnel: [u8 1 ("Slave ID") u8 2 ("Slave ID") u8 3 ("Slave ID") u8 4 ("Slave ID")] -> w1024
          frame "氨氮停止", Default {
          }
          frame "总氮停止", "总磷停止" {
          }
          frame "CODMn停止" {
          }
          frame "CODCr模块" {
          }
        }
        n660 = call "单个写入.vi"("value"=u16 2, "address"=u16 103, "Slave ID"=w1024) -> ()  [unwired: 8 in, 1 out]
      }
      event "氨氮排液", "CODMn排液", "总磷排液", "总氮排液", "CODCr排液": Value Change {
        n661 = event-data() -> ("CtlRef"=w1037:refnum<vi>)  [unwired: 1 in, 5 out]
        n662 = property class="Bool"(reference=w1037) -> ("Label.Text"=w1036:string)  [unwired: 1 in, 2 out]
        n663 = case shown="\"CODCr模块\"" w1036 {
          tunnel: [u8 1 ("Slave ID") u8 2 ("Slave ID") u8 3 ("Slave ID") u8 4 ("Slave ID")] -> w1033
          frame "氨氮排液", Default {
          }
          frame "总氮排液", "总磷排液" {
          }
          frame "CODMn排液" {
          }
          frame "CODCr模块" {
          }
        }
        n664 = call "单个写入.vi"("value"=u16 3, "address"=u16 103, "Slave ID"=w1033) -> ()  [unwired: 8 in, 1 out]
      }
      event "加标回收": Value Change {
        n665 = event-data() -> ()  [unwired: 1 in, 6 out]
        n666 = flat-sequence {
          tunnel: [w1046] -> w1045
          tunnel: [w1050] -> w1044
          tunnel: [w1049] -> w1043
          tunnel: w1042 -> [w1047]
          tunnel: w1045 -> [w1058]
          tunnel: w1044 -> [w1057]
          tunnel: w1043 -> [w1056]
          frame #0 {
            n667 = Send Notification(notification=FALSE ("通知"), notifier=w1047) -> ()  [unwired: 1 in, 2 out]
            n668 = call "质控启动流程对话框.vi"() -> ("启动模块"=w1046:T15, "直接启动"=w1049:bool, "常规启动"=w1050:bool)  [unwired: 8 in, 1 out]
            "常规启动" <- w1050
            "直接启动" <- w1049
          }
          frame #1 {
            n669 = Bundle By Name(cluster=T12 {"是否启用仪器"=FALSE, "CODMn"={"启动测量模式"={"测量模式"=enum."水样测量"}, "确定按钮"=FALSE}, "启动模块"={"氨氮"=FALSE, "总磷"=FALSE, "总氮"=FALSE, "CODMn"=FALSE, "CODCr"=FALSE}, "常规启动"=FALSE, "直接启动"=FALSE} ("参数"), "是否启用仪器"=TRUE, "启动模块"=w1058, "常规启动"=w1057, "直接启动"=w1056) -> (w1051:T12)
            n670 = vi-ref "质控单元.lvlib:一体站流程质控自动启动.vi"() -> (w1054:refnum<vi>)
            n671 = property class="VI"(reference=w1054) -> ("Name"=w1055:string, "Exec.State"=w1053:T16)  [unwired: 1 in, 2 out]
            n672 = case shown="\"Idle\"" w1053 {
              tunnel: w1055 -> [_ w1070]
              tunnel: w1051 -> [_ w1060]
              frame "Bad", Default {
              }
              frame "Idle" {
                n673 = Open VI Reference(type specifier VI Refnum (for type only)=refnum<vi> refnum ("类型说明符VI引用句柄（仅用于类型）"), vi path=w1070, options=128 ("选项")) -> (vi reference=w1071:refnum<vi>, error out=w1067:errorcluster)  [unwired: 3 in]
                n674 = call-by-ref "开始异步调用"(reference=w1071, error in=w1067, "CODMn量程切换"="CODMn量程选择", "总磷量程切换"="总磷量程选择", "总氮量程切换"="总氮量程选择", "氨氮量程切换"="氨氮量程选择", "参数"=w1060) -> (reference out=w1069:refnum<vi>, error out=w1068:errorcluster)  [unwired: 7 in]
                n675 = Close Reference(reference=w1069, error in (no error)=w1068) -> ()  [unwired: 1 out]
              }
            }
          }
        }
      }
      event "报警清除": Value Change {
        w1078 = FALSE ("氨氮中断报警")
        n676 = event-data() -> ()  [unwired: 1 in, 6 out]
        n677 = local read "氨氮模块"() -> (w1088:bool)
        n678 = local read "氨氮模块"() -> (w1079:bool)
        n679 = case shown="真" w1088 {
          tunnel: [errorcluster {"status"=FALSE, "code"=0, "source"=""} ("error out") w1131] -> w1085
          frame False {
          }
          frame True {
            n680 = call "多个线圈写入.vi"("values"=bool[] [TRUE], "starting address"=u16 2106, "Slave ID"=u8 1) -> ("error out"=w1131:errorcluster)  [unwired: 8 in]
          }
        }
        n681 = local read "总磷总氮模块选择"() -> (w1087:bool)
        n682 = local read "总磷总氮模块选择"() -> (w1080:bool)
        n683 = case shown="真" w1087 {
          tunnel: w1085 -> [w1124 w1127]
          tunnel: [w1124 w1125] -> w1084
          frame False {
          }
          frame True {
            n684 = call "多个线圈写入.vi"("Error in"=w1127, "values"=bool[] [TRUE], "starting address"=u16 2106, "Slave ID"=u8 2) -> ("error out"=w1125:errorcluster)  [unwired: 7 in]
          }
        }
        n685 = local read "CODMn选择"() -> (w1086:bool)
        n686 = local read "CODMn选择"() -> (w1081:bool)
        n687 = case shown="真" w1086 {
          tunnel: w1084 -> [w1118 w1122]
          tunnel: [w1118 w1119] -> w1075
          frame False {
          }
          frame True {
            n688 = call "多个线圈写入.vi"("Error in"=w1122, "values"=bool[] [TRUE], "starting address"=u16 2106, "Slave ID"=u8 3) -> ("error out"=w1119:errorcluster)  [unwired: 7 in]
          }
        }
        n689 = global write "质控中断报警全局.vi" "CODMn中断报警"(w1078) -> ()
        n690 = global write "质控中断报警全局.vi" "氨氮中断报警"(w1078) -> ()
        n691 = global write "质控中断报警全局.vi" "CODCr中断报警"(w1078) -> ()
        n692 = global write "质控中断报警全局.vi" "总氮中断报警"(w1078) -> ()
        n693 = global write "质控中断报警全局.vi" "总磷中断报警"(w1078) -> ()
        n694 = local read "CODCr选择"() -> (w1076:bool)
        n695 = local read "CODCr选择"() -> (w1077:bool)
        n696 = case shown="真" w1076 {
          tunnel: w1075 -> [w1095 w1099]
          tunnel: [w1095 w1096] -> w1074
          frame False {
          }
          frame True {
            n697 = call "多个线圈写入.vi"("Error in"=w1099, "values"=bool[] [TRUE], "starting address"=u16 2106, "Slave ID"=u8 4) -> ("error out"=w1096:errorcluster)  [unwired: 7 in]
          }
        }
        n698 = case shown="假" w1079 {
          tunnel: [w1113 w1114] -> w1082
          tunnel: w1074 -> [w1113 _]
          frame False {
          }
          frame True {
            n699 = call "多个线圈写入.vi"("values"=bool[] [FALSE], "starting address"=u16 2106, "Slave ID"=u8 1) -> ("error out"=w1114:errorcluster)  [unwired: 8 in]
          }
        }
        n700 = case shown="真" w1080 {
          tunnel: w1082 -> [w1107 w1110]
          tunnel: [w1107 w1108] -> w1083
          frame False {
          }
          frame True {
            n701 = call "多个线圈写入.vi"("Error in"=w1110, "values"=bool[] [FALSE], "starting address"=u16 2106, "Slave ID"=u8 2) -> ("error out"=w1108:errorcluster)  [unwired: 7 in]
          }
        }
        n702 = case shown="真" w1081 {
          tunnel: w1083 -> [w1101 w1105]
          tunnel: [w1101 w1102] -> w1073
          frame False {
          }
          frame True {
            n703 = call "多个线圈写入.vi"("Error in"=w1105, "values"=bool[] [FALSE], "starting address"=u16 2106, "Slave ID"=u8 3) -> ("error out"=w1102:errorcluster)  [unwired: 7 in]
          }
        }
        n704 = case shown="真" w1077 {
          tunnel: w1073 -> [w1089 w1093]
          tunnel: [w1089 w1090] -> w1072
          frame False {
          }
          frame True {
            n705 = call "多个线圈写入.vi"("Error in"=w1093, "values"=bool[] [FALSE], "starting address"=u16 2106, "Slave ID"=u8 4) -> ("error out"=w1090:errorcluster)  [unwired: 7 in]
          }
        }
      }
      event "氨氮加标回收启动": Value Change {
        n706 = event-data() -> ()  [unwired: 1 in, 6 out]
        n707 = Two Button Dialog(message="确定启动氨氮的加标回收？" ("消息"), 1:"否" ("F按钮名称（“取消”）"), 2:"是" ("T按钮名称（“确定”）")) -> (T button?=w1135:bool)
        n708 = case shown="真" w1135 {
          frame False {
          }
          frame True {
            n709 = vi-ref "质控单元.lvlib:氨氮流程质控自动启动.vi"() -> (w1141:refnum<vi>)
            n710 = property class="VI"(reference=w1141) -> ("Name"=w1139:string, "Exec.State"=w1140:T16)  [unwired: 1 in, 2 out]
            n711 = case shown="\"Idle\"" w1140 {
              tunnel: w1139 -> [_ w1145 _ _]
              frame "Bad", Default {
              }
              frame "Idle" {
                n712 = local read "氨氮量程选择"() -> (w1144:enum32{"H", "L", "AUTO"})
                n713 = Open VI Reference(type specifier VI Refnum (for type only)=refnum<vi> refnum ("类型说明符VI引用句柄（仅用于类型）"), vi path=w1145, options=128 ("选项")) -> (vi reference=w1149:refnum<vi>, error out=w1143:errorcluster)  [unwired: 3 in]
                n714 = call-by-ref "开始异步调用"(reference=w1149, error in=w1143, "氨氮量程切换"=w1144) -> (reference out=w1148:refnum<vi>, error out=w1142:errorcluster)  [unwired: 11 in]
                n715 = Close Reference(reference=w1148, error in (no error)=w1142) -> ()  [unwired: 1 out]
              }
              frame "Run top level" {
              }
              frame "Running" {
              }
            }
          }
        }
      }
      event "总磷总氮加标回收启动": Value Change {
        w1152 = TRUE ("总氮")
        w1153 = FALSE ("氨氮")
        n716 = event-data() -> ()  [unwired: 1 in, 6 out]
        n717 = call "质控启动参数选择对话框.vi"("COD"=w1153, "总氮"=w1152, "总磷"=w1152, "氨氮"=w1153) -> ("确定启动"=w1151:bool, "启动模块"=w1150:T15)  [unwired: 5 in, 1 out]
        n718 = case shown="真" w1151 {
          tunnel: w1150 -> [_ w1156]
          frame False {
          }
          frame True {
            n719 = vi-ref "质控单元.lvlib:总磷总氮流程质控自动启动.vi"() -> (w1159:refnum<vi>)
            n720 = Unbundle By Name(w1156) -> ("总磷"=w1155:bool, "总氮"=w1154:bool)
            n721 = property class="VI"(reference=w1159) -> ("Name"=w1157:string, "Exec.State"=w1158:T16)  [unwired: 1 in, 2 out]
            n722 = case shown="\"Idle\"" w1158 {
              tunnel: w1157 -> [_ w1168 _ _]
              tunnel: w1155 -> [_ w1161 _ _]
              tunnel: w1154 -> [_ w1160 _ _]
              frame "Bad", Default {
              }
              frame "Idle" {
                n723 = Bundle By Name(cluster=T13 {"是否启用仪器"=FALSE, "CODMn"={"启动测量模式"={"测量模式"=enum."水样测量"}, "确定按钮"=FALSE}, "启动模块"={"氨氮"=FALSE, "总磷"=FALSE, "总氮"=FALSE, "COD"=FALSE}, "常规启动"=FALSE, "直接启动"=FALSE} ("参数"), "启动模块.总磷"=w1161, "启动模块.总氮"=w1160) -> (w1162:T13)
                n724 = local read "总氮量程选择"() -> (w1165:enum32{"H", "L", "AUTO"})
                n725 = local read "总磷量程选择"() -> (w1164:enum32{"H", "L", "AUTO"})
                n726 = Open VI Reference(type specifier VI Refnum (for type only)=refnum<vi> refnum ("类型说明符VI引用句柄（仅用于类型）"), vi path=w1168, options=128 ("选项")) -> (vi reference=w1172:refnum<vi>, error out=w1166:errorcluster)  [unwired: 3 in]
                n727 = call-by-ref "开始异步调用"(reference=w1172, error in=w1166, "总磷量程切换"=w1164, "总氮量程切换"=w1165, "参数"=w1162) -> (reference out=w1171:refnum<vi>, error out=w1167:errorcluster)  [unwired: 9 in]
                n728 = Close Reference(reference=w1171, error in (no error)=w1167) -> ()  [unwired: 1 out]
              }
              frame "Run top level" {
              }
              frame "Running" {
              }
            }
          }
        }
      }
      event "CODMn加标回收启动": Value Change {
        n729 = event-data() -> ()  [unwired: 1 in, 6 out]
        n730 = Two Button Dialog(message="确定启动CODMn的加标回收？" ("消息"), 1:"否" ("F按钮名称（“取消”）"), 2:"是" ("T按钮名称（“确定”）")) -> (T button?=w1173:bool)
        n731 = case shown="真" w1173 {
          frame False {
          }
          frame True {
            n732 = vi-ref "CODMn流程质控自动启动.vi"() -> (w1179:refnum<vi>)
            n733 = property class="VI"(reference=w1179) -> ("Name"=w1177:string, "Exec.State"=w1178:T16)  [unwired: 1 in, 2 out]
            n734 = case shown="\"Idle\"" w1178 {
              tunnel: w1177 -> [_ w1183 _ _]
              frame "Bad", Default {
              }
              frame "Idle" {
                n735 = local read "CODMn量程选择"() -> (w1180:enum32{"H", "L", "AUTO"})
                n736 = Open VI Reference(type specifier VI Refnum (for type only)=refnum<vi> refnum ("类型说明符VI引用句柄（仅用于类型）"), vi path=w1183, options=128 ("选项")) -> (vi reference=w1187:refnum<vi>, error out=w1182:errorcluster)  [unwired: 3 in]
                n737 = call-by-ref "开始异步调用"(reference=w1187, error in=w1182, "CODMn量程切换"=w1180) -> (reference out=w1186:refnum<vi>, error out=w1181:errorcluster)  [unwired: 10 in]
                n738 = Close Reference(reference=w1186, error in (no error)=w1181) -> ()  [unwired: 1 out]
              }
              frame "Run top level" {
              }
              frame "Running" {
              }
            }
          }
        }
      }
      event "CODCr加标回收启动": Value Change {
        n739 = event-data() -> ()  [unwired: 1 in, 6 out]
        n740 = Two Button Dialog(message="确定启动CODCr的加标回收？" ("消息"), 1:"否" ("F按钮名称（“取消”）"), 2:"是" ("T按钮名称（“确定”）")) -> (T button?=w1188:bool)
        n741 = case shown="真" w1188 {
          frame False {
          }
          frame True {
            n742 = vi-ref "CODCr流程质控自动启动.vi"() -> (w1194:refnum<vi>)
            n743 = property class="VI"(reference=w1194) -> ("Name"=w1192:string, "Exec.State"=w1193:T16)  [unwired: 1 in, 2 out]
            n744 = case shown="\"Idle\"" w1193 {
              tunnel: w1192 -> [_ w1198 _ _]
              frame "Bad", Default {
              }
              frame "Idle" {
                n745 = local read "CODCr量程选择"() -> (w1195:enum32{"H", "L", "AUTO"})
                n746 = Open VI Reference(type specifier VI Refnum (for type only)=refnum<vi> refnum ("类型说明符VI引用句柄（仅用于类型）"), vi path=w1198, options=128 ("选项")) -> (vi reference=w1202:refnum<vi>, error out=w1197:errorcluster)  [unwired: 3 in]
                n747 = call-by-ref "开始异步调用"(reference=w1202, error in=w1197, "CODMn量程切换"=w1195) -> (reference out=w1201:refnum<vi>, error out=w1196:errorcluster)  [unwired: 10 in]
                n748 = Close Reference(reference=w1201, error in (no error)=w1196) -> ()  [unwired: 1 out]
              }
              frame "Run top level" {
              }
              frame "Running" {
              }
            }
          }
        }
      }
      event "平行样测试": Value Change {
        n749 = event-data() -> ()  [unwired: 1 in, 6 out]
        n750 = flat-sequence {
          tunnel: [w1208] -> w1206
          tunnel: [w1210] -> w1205
          tunnel: [w1209] -> w1204
          tunnel: w1203 -> [w1207]
          tunnel: w1206 -> [w1217]
          tunnel: w1205 -> [w1216]
          tunnel: w1204 -> [w1215]
          frame #0 {
            n751 = Cancel Notification(0:w1207) -> ()  [unwired: 1 in, 3 out]
            n752 = call "平行样启动流程对话框.vi"() -> ("启动模块"=w1208:cluster{"氨氮1":bool, "总磷1":bool, " COD1":bool}, "直接启动"=w1209:bool, "常规启动"=w1210:bool)  [unwired: 8 in, 1 out]
            "常规启动 2" <- w1210
            "直接启动 2" <- w1209
            "启动模块 2" <- w1208
          }
          frame #1 {
            n753 = Bundle By Name(cluster=T4 {"是否启用仪器"=FALSE, "CODMn"={"启动测量模式"={"测量模式"=enum."水样测量"}, "确定按钮"=TRUE}, "启动模块"={"氨氮1"=FALSE, "总磷1"=FALSE, " COD1"=FALSE}, "常规启动"=FALSE, "直接启动"=FALSE} ("参数"), "是否启用仪器"=TRUE, "启动模块"=w1217, "常规启动"=w1216, "直接启动"=w1215) -> (w1212:T4)
            "输出簇 2" <- w1212
            n754 = vi-ref "一体站流程平行样自动启动.vi"() -> (w1213:refnum<vi>)
            n755 = property class="VI"(reference=w1213) -> ("Name"=w1214:string, "Exec.State"=w1211:T16)  [unwired: 1 in, 2 out]
            n756 = case shown="\"Idle\"" w1211 {
              tunnel: w1214 -> [_ w1226]
              tunnel: w1212 -> [_ w1220]
              frame "Bad", Default {
              }
              frame "Idle" {
                n757 = Open VI Reference(type specifier VI Refnum (for type only)=refnum<vi> refnum ("类型说明符VI引用句柄（仅用于类型）"), vi path=w1226, options=128 ("选项")) -> (vi reference=w1227:refnum<vi>, error out=w1225:errorcluster)  [unwired: 3 in]
                n758 = call-by-ref "开始异步调用"(reference=w1227, error in=w1225, "参数"=w1220) -> (reference out=w1222:refnum<vi>, error out=w1221:errorcluster)  [unwired: 9 in]
                n759 = Close Reference(reference=w1222, error in (no error)=w1221) -> ()  [unwired: 1 out]
              }
            }
          }
        }
      }
      event "停止测量": Value Change {
        w1228 = TRUE ("氨氮")
        # "停止采配水、氨氮、总磷总氮、COD、质控"
        n760 = event-data() -> ()  [unwired: 1 in, 6 out]
        n761 = call "质控启动参数选择对话框.vi"("COD"=w1228, "总氮"=w1228, "总磷"=w1228, "氨氮"=w1228) -> ("确定启动"=w1229:bool, "启动模块"=w1230:T15)  [unwired: 5 in, 1 out]
        n762 = case shown="真" w1229 {
          tunnel: w1230 -> [_ w1240]
          frame False {
          }
          frame True {
            n763 = Unbundle By Name(w1240) -> ("氨氮"=w1238:bool, "总磷"=w1237:bool, "总氮"=w1236:bool, "CODMn"=w1239:bool)
            n764 = Or(x=w1237, y=w1236) -> (x .or. y?=w1235:bool)
            n765 = case shown="真" w1239 {
              frame False {
              }
              frame True {
                n766 = call "CODMn停止命令 (子VI).vi"() -> ()  [unwired: 12 in]
                n767 = Obtain Notifier(name (unnamed)="CODMn" ("名称（未命名）"), notification data type=FALSE) -> (notifier out=w1266:refnum<notifier>)  [unwired: 2 in, 2 out]
                n768 = Send Notification(notification=TRUE ("通知"), notifier=w1266) -> ()  [unwired: 1 in, 2 out]
                n769 = call "单个写入.vi"("value"=u16 2, "address"=u16 103, "Slave ID"=u8 3) -> ()  [unwired: 8 in, 1 out]
              }
            }
            n770 = case shown="真" w1238 {
              frame False {
              }
              frame True {
                n771 = Obtain Queue(name (unnamed)="NH3N" ("名称（未命名）"), element data type=cluster{"命令":string, "data":variant} {"命令"="", "data"=variant}) -> (queue out=w1262:refnum<queue>)  [unwired: 3 in, 2 out]
                n772 = Enqueue Element(queue=w1262, element=cluster{"命令":string, "data":variant} {"命令"="启动", "data"=variant(cluster{"站号":u16, "控制命令输出":u16[]} {"站号"=1, "控制命令输出"=[2816]})} ("元素")) -> ()  [unwired: 2 in, 3 out]
                n773 = Obtain Notifier(name (unnamed)="NH3N" ("名称（未命名）"), notification data type=FALSE) -> (notifier out=w1258:refnum<notifier>)  [unwired: 2 in, 2 out]
                n774 = Send Notification(notification=TRUE ("通知"), notifier=w1258) -> ()  [unwired: 1 in, 2 out]
                n775 = call "单个写入.vi"("value"=u16 2, "address"=u16 103, "Slave ID"=u8 1) -> ()  [unwired: 8 in, 1 out]
              }
            }
            n776 = case shown="真" w1235 {
              frame False {
              }
              frame True {
                n777 = Obtain Queue(name (unnamed)="TP" ("名称（未命名）"), element data type=cluster{"命令":string, "data":variant} {"命令"="", "data"=variant}) -> (queue out=w1251:refnum<queue>)  [unwired: 3 in, 2 out]
                n778 = Enqueue Element(queue=w1251, element=cluster{"命令":string, "data":variant} {"命令"="启动", "data"=variant(cluster{"站号":u16, "控制命令输出":u16[]} {"站号"=1, "控制命令输出"=[2816]})} ("元素")) -> ()  [unwired: 2 in, 3 out]
                n779 = Obtain Notifier(name (unnamed)="TNTP" ("名称（未命名）"), notification data type=FALSE) -> (notifier out=w1247:refnum<notifier>)  [unwired: 2 in, 2 out]
                n780 = Send Notification(notification=TRUE ("通知"), notifier=w1247) -> ()  [unwired: 1 in, 2 out]
                n781 = call "单个写入.vi"("value"=u16 2, "address"=u16 103, "Slave ID"=u8 2) -> ()  [unwired: 8 in, 1 out]
              }
            }
          }
        }
        n782 = Send Notification(notification=TRUE ("通知"), notifier=w1234) -> ()  [unwired: 1 in, 2 out]
        n783 = Enqueue Element At Opposite End(queue=w1231, element=T14 {"命令"="单个写入", {"starting address"=300, "holding register value"=2}} ("元素")) -> ()  [unwired: 2 in, 3 out]
      }
      event "查看": Value Change {
        n784 = event-data() -> ()  [unwired: 1 in, 6 out]
        n785 = property on="窗格" class="Pane"("Origin"=T5 {"Horizontal"=0, "Vertical"=600} ("原点")) -> ()  [unwired: 2 in, 2 out]
      }
      event "返回": Value Change {
        n786 = event-data() -> ()  [unwired: 1 in, 6 out]
        n787 = property on="窗格" class="Pane"("Origin"=T5 {"Horizontal"=0, "Vertical"=0} ("原点")) -> ()  [unwired: 2 in, 2 out]
      }
    }
  }
  n788 = call "质控参数读取.vi"("section"="CODCr质控参数", "error in (no error)"=w18) -> ("参数"=w19:T6)  [unwired: 8 in, 1 out]
  n789 = Unbundle By Name(w19) -> ("量程"=→"CODCr量程":dbl, "检出限"=→"CODCr检出限":dbl, "加标前水样浓度"=→"CODCr加标前水样浓度":dbl, "加标后水样浓度"=→"CODCr加标后水样浓度":dbl, "加标水杯定容体积"=→"CODCr加标水杯定容体积":dbl, "加标母液浓度"=→"CODCr母液浓度":dbl, "加标体积"=→"CODCr加标体积":dbl, "加标回收率"=→"CODCr加标回收率":dbl)
  n790 = call-dynamic "Close Session.vi"("error in (no error)"=w53, "MB_Serial session"=w23) -> ()  [unwired: 9 in, 1 out]
  "VISA Resource" <- w22
  "Serial Config" <- w21
